vi "RSZVB VI Tree.vi"   [LabVIEW 2011]
doc: "This is the instrument driver for the R&S ZVB Network Analyzer. The VI Tree displays all the user-callable VIs of the instrument driver in an organized table.\n\nInstrument Driver Name: ZVB Network Analyzer\nInstrument Manufacturer: Rohde & Schwarz\nInstrument Type: Network Analyzer\nSupported Models: ZVB Series\nSupported Bus Types: IEEE 488.2 (IEC-625, GPIB), RSIB, VXI-11\n\nInstrument Driver Version: 3.40.0\nSupported Firmware: 3.40\nCreated By: Martin Koutny\nRelease Date: September 2004\nOriginally Developed in LabVIEW Version: 6.1\nOriginally Developed using VISA Version: 3.0.1\n\nUnsupported Instrument Features: none\n\nFor detailed driver information including modification history, refer to the <B>RSZVB.chm </B> file."
panel:
  # "SEE DIAGRAM\nFOR VI TREE."
diagram:
  # "ZVAX-TRM Extension Unit"
  # "Simultaneous Measurement"
  # "Universal Interface"
  # "Get Source Power Calibration Parameters"
  # "Renormalization"
  # "Noise Figure"
  # "Source Power Calibration"
  # "Converter"
  # "Power Port Limits"
  # "PI Controller Low-Level"
  # "Define Port Pair"
  # "Bandwidth Fine Adjust"
  # "Noise Figure"
  # "Low-Level"
  # "Linearity Deviation"
  # "Low Level"
  # "ZVAX Path Configuration"
  # "Low Level"
  # "Pulse Generator"
  # "ZVAX24 Extension Unit"
  # "Fixture Compensation"
  # "Vector Mixer Measurement"
  # "Mixer Delay"
  # "Max Min Hold On"
  # "Defined Coherence Mode"
  # "Intermodulation Distortion"
  # "Multiport Config"
  # "Define Ripple Test"
  # "Ripple"
  # "Power Meter"
  # "True Differential Mode"
  # "Time Out"
  # "Loss Low-Level"
  # "Stimulus"
  # "Pulsed Measurement"
  # "Virtual Transform"
  # "Receiver Power Calibration"
  # "Low-Level"
  # "Modify Source Power Calibration"
  # "Source Power Calibration"
  # "Power Calibration"
  # "Mixer Power Calibration"
  # "Low-Level"
  # "Set Frequencies"
  # "Low-Level"
  # "Set Powers"
  # "Define Mixer Measurement"
  # "Mixer"
  # "System Softkeys"
  # "Low-Level"
  # "Harmonic Distortion"
  # "Define Time Gate"
  # "Low Pass Settings"
  # "Define Transform"
  # "Time Domain Stimulus"
  # "Transform"
  # "Sweep"
  # "Low-Level"
  # "Sweep Time"
  # "Trace Shift"
  # "Import (Export) Data"
  # "Trace Data"
  # "Trace Smoothing"
  # "Trace Evaluation"
  # "User Defined Math"
  # "Define Limit Line(s)"
  # "Status Subsystem"
  # "Initialize"
  # "Close"
  # "Application Example"
  # "Getting Started"
  # "Utility"
  # "Reference"
  # "Channel Bits"
  # "System Config"
  # "System"
  # "Config (View)"
  # "Area Select"
  # "Display"
  # "Mechanical Length Low-Level"
  # "Offset"
  # "Calibration Kits"
  # "Calibration Lists"
  # "Connectors"
  # "Calibration"
  # "Channel Select"
  # "Low-Level"
  # "SAW Matching Network"
  # "Reference Impedances"
  # "Define Balanced Port"
  # "Define Measured Ports"
  # "Port Config"
  # "Mode"
  # "Low-Level"
  # "Trigger"
  # "Define Segments"
  # "Sweep Type"
  # "Low-Level"
  # "Power Bandwidth Average"
  # "Stimulus"
  # "Channel"
  # "Lines"
  # "Marker Funct(ions)"
  # "Bandfilter Search"
  # "Target Search"
  # "Search"
  # "Marker"
  # "Trace Funct(ions)"
  # "Trace Select"
  # "Scale"
  # "Format"
  # "DC Inputs"
  # "Stability Factor"
  # "Y-Parameters"
  # "Z-Parameters"
  # "Admittance"
  # "Impedance"
  # "Wave Quantities"
  # "Ratios"
  # "S-Parameters"
  # "Measure"
  # "Trace"
  # "File (Mass Storage Capabilities)"
  # "Print"
  # "Window Select"
  # "File"
  # "R&S ZVB Network Analyzer"
  n1 = call "RSZVB Set Power Port Limit State.vi"() -> ()  [unwired: 10 in, 2 out]
  n2 = call "RSZVB Set Presets.vi"() -> ()  [unwired: 10 in, 2 out]
  n3 = call "RSZVB Set User Defined Preset State.vi"() -> ()  [unwired: 10 in, 2 out]
  n4 = call "RSZVB Set Display Update.vi"() -> ()  [unwired: 10 in, 2 out]
  n5 = call "RSZVB Get Remote Language.vi"() -> ()  [unwired: 9 in, 3 out]
  n6 = call "RSZVB Configure External Power Meter.vi"() -> ()  [unwired: 10 in, 2 out]
  n7 = call "RSZVB Get Auto Config NRPZxx.vi"() -> ()  [unwired: 9 in, 3 out]
  n8 = call "RSZVB Set Frequency Conversion Type.vi"() -> ()  [unwired: 10 in, 2 out]
  n9 = call "RSZVB Set Power Coeficients.vi"() -> ()  [unwired: 10 in, 2 out]
  n10 = call "RSZVB Set NWA Application Priority.vi"() -> ()  [unwired: 10 in, 2 out]
  n11 = call "RSZVB Set RF Off Behavior.vi"() -> ()  [unwired: 10 in, 2 out]
  n12 = call "RSZVB Set Soft Key Label.vi"() -> ()  [unwired: 10 in, 2 out]
  n13 = call "RSZVB Set Reference.vi"() -> ()  [unwired: 10 in, 2 out]
  n14 = call "RSZVB Set Status Register.vi"() -> ()  [unwired: 10 in, 2 out]
  n15 = call "RSZVB Set Status Sounds State.vi"() -> ()  [unwired: 10 in, 2 out]
  n16 = call "RSZVB Set Output Port Bits.vi"() -> ()  [unwired: 10 in, 2 out]
  n17 = call "RSZVB Set UI Direction.vi"() -> ()  [unwired: 10 in, 2 out]
  n18 = call "RSZVB Set UI Signal Pin 21.vi"() -> ()  [unwired: 10 in, 2 out]
  n19 = call "RSZVB Restore UI Default States.vi"() -> ()  [unwired: 10 in, 2 out]
  n20 = call "RSZVB Reset Offsets.vi"() -> ()  [unwired: 10 in, 2 out]
  n21 = call "RSZVB Configure Loss.vi"() -> ()  [unwired: 10 in, 2 out]
  n22 = call "RSZVB Set Delay.vi"() -> ()  [unwired: 10 in, 2 out]
  n23 = call "RSZVB Set Font Size.vi"() -> ()  [unwired: 10 in, 2 out]
  n24 = call "RSZVB Set RGB Color.vi"() -> ()  [unwired: 10 in, 2 out]
  n25 = call "RSZVB Channel Add.vi"() -> ()  [unwired: 10 in, 2 out]
  n26 = call "RSZVB Channel Get Channel Name.vi"() -> ()  [unwired: 9 in, 3 out]
  n27 = call "RSZVB Diagram Area Add.vi"() -> ()  [unwired: 10 in, 2 out]
  n28 = call "RSZVB Set Color Scheme.vi"() -> ()  [unwired: 10 in, 2 out]
  n29 = call "RSZVB Set Ripple Check On.vi"() -> ()  [unwired: 10 in, 2 out]
  n30 = call "RSZVB Get Ripple Limit Check Segment Result.vi"() -> ()  [unwired: 8 in, 4 out]
  n31 = call "RSZVB Get Number Ripple Limit Ranges.vi"() -> ()  [unwired: 9 in, 3 out]
  n32 = call "RSZVB Set Marker State.vi"() -> ()  [unwired: 10 in, 2 out]
  n33 = call "RSZVB Set Reference Marker State.vi"() -> ()  [unwired: 10 in, 2 out]
  n34 = call "RSZVB Set Reference Discrete Marker.vi"() -> ()  [unwired: 10 in, 2 out]
  n35 = call "RSZVB Get Delta Marker State.vi"() -> ()  [unwired: 9 in, 3 out]
  n36 = call "RSZVB Set Fixed Marker.vi"() -> ()  [unwired: 10 in, 2 out]
  n37 = call "RSZVB Save All Markers.vi"() -> ()  [unwired: 10 in, 2 out]
  n38 = call "RSZVB Trace Get Trace Name.vi"() -> ()  [unwired: 9 in, 3 out]
  n39 = call "RSZVB Set Marker Tracking.vi"() -> ()  [unwired: 10 in, 2 out]
  n40 = call "RSZVB Set Limit Response Domain Format Units.vi"() -> ()  [unwired: 10 in, 2 out]
  n41 = call "RSZVB Window New.vi"() -> ()  [unwired: 10 in, 2 out]
  n42 = call "RSZVB Print.vi"() -> ()  [unwired: 10 in, 2 out]
  n43 = call "RSZVB File Manager.vi"() -> ()  [unwired: 10 in, 2 out]
  n44 = call "RSZVB Setup Recall.vi"() -> ()  [unwired: 10 in, 2 out]
  n45 = call "RSZVB Set Trace Format.vi"() -> ()  [unwired: 10 in, 2 out]
  n46 = call "RSZVB Trace Add.vi"() -> ()  [unwired: 10 in, 2 out]
  n47 = call "RSZVB Trace Add Diagram Area.vi"() -> ()  [unwired: 10 in, 2 out]
  n48 = call "RSZVB Trace Delete All.vi"() -> ()  [unwired: 10 in, 2 out]
  n49 = call "RSZVB Trace Data To Memory.vi"() -> ()  [unwired: 10 in, 2 out]
  n50 = call "RSZVB Marker Search.vi"() -> ()  [unwired: 10 in, 2 out]
  n51 = call "RSZVB Set Start To Marker.vi"() -> ()  [unwired: 10 in, 2 out]
  n52 = call "RSZVB Show Limit Line.vi"() -> ()  [unwired: 10 in, 2 out]
  n53 = call "RSZVB Set Limit Line TTL Out Pass 1(2).vi"() -> ()  [unwired: 10 in, 2 out]
  n54 = call "RSZVB Set Start Frequency.vi"() -> ()  [unwired: 10 in, 2 out]
  n55 = call "RSZVB Set Frequency Span.vi"() -> ()  [unwired: 10 in, 2 out]
  n56 = call "RSZVB Set Start Power.vi"() -> ()  [unwired: 10 in, 2 out]
  n57 = call "RSZVB Configure Power Bandwidth Average.vi"() -> ()  [unwired: 10 in, 2 out]
  n58 = call "RSZVB Get Trace Ref Position.vi"() -> ()  [unwired: 9 in, 3 out]
  n59 = call "RSZVB Trace Autoscale.vi"() -> ()  [unwired: 10 in, 2 out]
  n60 = call "RSZVB Get Trace Scale Divisions.vi"() -> ()  [unwired: 9 in, 3 out]
  n61 = call "RSZVB Create Trace.vi"() -> ()  [unwired: 10 in, 2 out]
  n62 = call "RSZVB Set Loss At DC.vi"() -> ()  [unwired: 10 in, 2 out]
  n63 = call "RSZVB Get Delay.vi"() -> ()  [unwired: 9 in, 3 out]
  n64 = call "RSZVB Acquire Fixture Compensation Sweep.vi"() -> ()  [unwired: 10 in, 2 out]
  n65 = call "RSZVB Set Fixture Compensation Direct Compensation.vi"() -> ()  [unwired: 10 in, 2 out]
  n66 = call "RSZVB Get Power Port Limit State.vi"() -> ()  [unwired: 9 in, 3 out]
  n67 = call "RSZVB Get Presets.vi"() -> ()  [unwired: 9 in, 3 out]
  n68 = call "RSZVB Get Display Update.vi"() -> ()  [unwired: 9 in, 3 out]
  n69 = call "RSZVB Configure External Generator.vi"() -> ()  [unwired: 14 in, 2 out]
  n70 = call "RSZVB Query External Power Meter.vi"() -> ()  [unwired: 6 in, 6 out]
  n71 = call "RSZVB Delete External Power Meter.vi"() -> ()  [unwired: 10 in, 2 out]
  n72 = call "RSZVB Get Status Sounds State.vi"() -> ()  [unwired: 9 in, 3 out]
  n73 = call "RSZVB Get Frequency Conversion Type.vi"() -> ()  [unwired: 9 in, 3 out]
  n74 = call "RSZVB Get Power Coeficients.vi"() -> ()  [unwired: 9 in, 3 out]
  n75 = call "RSZVB Get NWA Application Priority.vi"() -> ()  [unwired: 9 in, 3 out]
  n76 = call "RSZVB Get RF Off Behavior.vi"() -> ()  [unwired: 9 in, 3 out]
  n77 = call "RSZVB Get Pressed Soft Key.vi"() -> ()  [unwired: 8 in, 4 out]
  n78 = call "RSZVB Get Output Port Bits.vi"() -> ()  [unwired: 9 in, 3 out]
  n79 = call "RSZVB Get UI Direction.vi"() -> ()  [unwired: 9 in, 3 out]
  n80 = call "RSZVB Get UI Signal Pin 21.vi"() -> ()  [unwired: 9 in, 3 out]
  n81 = call "RSZVB Get Reference.vi"() -> ()  [unwired: 9 in, 3 out]
  n82 = call "RSZVB Get Status Register.vi"() -> ()  [unwired: 9 in, 3 out]
  n83 = call "RSZVB Set Mechanical Length.vi"() -> ()  [unwired: 10 in, 2 out]
  n84 = call "RSZVB Get RGB Color.vi"() -> ()  [unwired: 5 in, 7 out]
  n85 = call "RSZVB Get User Defined Preset State.vi"() -> ()  [unwired: 9 in, 3 out]
  n86 = call "RSZVB Export Kit.vi"() -> ()  [unwired: 10 in, 2 out]
  n87 = call "RSZVB Channel Add Trace.vi"() -> ()  [unwired: 10 in, 2 out]
  n88 = call "RSZVB Channel Get Channel Number.vi"() -> ()  [unwired: 9 in, 3 out]
  n89 = call "RSZVB Set Connector.vi"() -> ()  [unwired: 10 in, 2 out]
  n90 = call "RSZVB Select Calibration Type.vi"() -> ()  [unwired: 14 in, 2 out]
  n91 = call "RSZVB Get Calibration Reference Plane Shift.vi"() -> ()  [unwired: 9 in, 3 out]
  n92 = call "RSZVB Delete Calibration Data.vi"() -> ()  [unwired: 10 in, 2 out]
  n93 = call "RSZVB Set Calibration Kit.vi"() -> ()  [unwired: 10 in, 2 out]
  n94 = call "RSZVB Calibration Kit Catalog With Label.vi"() -> ()  [unwired: 9 in, 3 out]
  n95 = call "RSZVB Load Calibration Kit.vi"() -> ()  [unwired: 14 in, 2 out]
  n96 = call "RSZVB Query Reset Offsets.vi"() -> ()  [unwired: 9 in, 3 out]
  n97 = call "RSZVB Diagram Area Delete.vi"() -> ()  [unwired: 10 in, 2 out]
  n98 = call "RSZVB Get Color Scheme.vi"() -> ()  [unwired: 9 in, 3 out]
  n99 = call "RSZVB Get Font Size.vi"() -> ()  [unwired: 9 in, 3 out]
  n100 = call "RSZVB Set User Connector.vi"() -> ()  [unwired: 10 in, 2 out]
  n101 = call "RSZVB Set Source Power Correction State.vi"() -> ()  [unwired: 10 in, 2 out]
  n102 = call "RSZVB Calibration Auto Simplified.vi"() -> ()  [unwired: 10 in, 2 out]
  n103 = call "RSZVB Calibration Auto Assignment Type.vi"() -> ()  [unwired: 10 in, 2 out]
  n104 = call "RSZVB Set Calibration Data Current State.vi"() -> ()  [unwired: 10 in, 2 out]
  n105 = call "RSZVB Set Calibration Connector.vi"() -> ()  [unwired: 10 in, 2 out]
  n106 = call "RSZVB Get Calibration Label.vi"() -> ()  [unwired: 9 in, 3 out]
  n107 = call "RSZVB Get Calibration Data Receiver Attenuation.vi"() -> ()  [unwired: 8 in, 4 out]
  n108 = call "RSZVB Get Active Calibration Unit.vi"() -> ()  [unwired: 9 in, 3 out]
  n109 = call "RSZVB Get Factory Calibration State.vi"() -> ()  [unwired: 9 in, 3 out]
  n110 = call "RSZVB Get Calibration Correction Base Frequency State.vi"() -> ()  [unwired: 9 in, 3 out]
  n111 = call "RSZVB Get Ripple Check On.vi"() -> ()  [unwired: 9 in, 3 out]
  n112 = call "RSZVB Set Ripple Limits Display State.vi"() -> ()  [unwired: 10 in, 2 out]
  n113 = call "RSZVB Add Ripple Limit Line Ranges Segment.vi"() -> ()  [unwired: 10 in, 2 out]
  n114 = call "RSZVB Set Ripple Limit Range.vi"() -> ()  [unwired: 10 in, 2 out]
  n115 = call "RSZVB Get Marker Tracking.vi"() -> ()  [unwired: 9 in, 3 out]
  n116 = call "RSZVB Set Sweep Number Of Points.vi"() -> ()  [unwired: 10 in, 2 out]
  n117 = call "RSZVB Configure Sweep Time.vi"() -> ()  [unwired: 10 in, 2 out]
  n118 = call "RSZVB Trace Add Mode.vi"() -> ()  [unwired: 10 in, 2 out]
  n119 = call "RSZVB Trace Assign Diagram Area.vi"() -> ()  [unwired: 10 in, 2 out]
  n120 = call "RSZVB Channel Trace Export Data With Options.vi"() -> ()  [unwired: 10 in, 2 out]
  n121 = call "RSZVB Set Coherent Signal Reference Port.vi"() -> ()  [unwired: 10 in, 2 out]
  n122 = call "RSZVB Trace Delete All Channels.vi"() -> ()  [unwired: 10 in, 2 out]
  n123 = call "RSZVB Trace Get Trace Number.vi"() -> ()  [unwired: 9 in, 3 out]
  n124 = call "RSZVB Trace Data To Memory Trace.vi"() -> ()  [unwired: 10 in, 2 out]
  n125 = call "RSZVB Get Marker State.vi"() -> ()  [unwired: 9 in, 3 out]
  n126 = call "RSZVB Get Reference Marker State.vi"() -> ()  [unwired: 9 in, 3 out]
  n127 = call "RSZVB Get Reference Discrete Marker.vi"() -> ()  [unwired: 9 in, 3 out]
  n128 = call "RSZVB Set Coupled Markers.vi"() -> ()  [unwired: 10 in, 2 out]
  n129 = call "RSZVB Get Fixed Marker.vi"() -> ()  [unwired: 9 in, 3 out]
  n130 = call "RSZVB Set Frequency Conversion.vi"() -> ()  [unwired: 14 in, 2 out]
  n131 = call "RSZVB Set Converter Source Frequency.vi"() -> ()  [unwired: 10 in, 2 out]
  n132 = call "RSZVB Set Local Oscilator B State.vi"() -> ()  [unwired: 10 in, 2 out]
  n133 = call "RSZVB Set Port Impedances Renormalization.vi"() -> ()  [unwired: 10 in, 2 out]
  n134 = call "RSZVB Set IF Gain Reference Channel.vi"() -> ()  [unwired: 10 in, 2 out]
  n135 = call "RSZVB Set Permanent Signal Generator State.vi"() -> ()  [unwired: 10 in, 2 out]
  n136 = call "RSZVB Set Source Combiner State.vi"() -> ()  [unwired: 10 in, 2 out]
  n137 = call "RSZVB Set TDIF State.vi"() -> ()  [unwired: 10 in, 2 out]
  n138 = call "RSZVB Get TDIF Amplitude Imbalance Start Power.vi"() -> ()  [unwired: 9 in, 3 out]
  n139 = call "RSZVB Set TDIF Phase Imbalance Start Phase.vi"() -> ()  [unwired: 10 in, 2 out]
  n140 = call "RSZVB Get TDIF Source Power Mode.vi"() -> ()  [unwired: 9 in, 3 out]
  n141 = call "RSZVB Set TRM Measure Input.vi"() -> ()  [unwired: 10 in, 2 out]
  n142 = call "RSZVB Get TRM Power Amplifier State.vi"() -> ()  [unwired: 9 in, 3 out]
  n143 = call "RSZVB Set TRM User Measurement Path Extension State.vi"() -> ()  [unwired: 10 in, 2 out]
  n144 = call "RSZVB Get TRM Pulse Generator Source.vi"() -> ()  [unwired: 9 in, 3 out]
  n145 = call "RSZVB Get TRM Unit Hardware Options.vi"() -> ()  [unwired: 9 in, 3 out]
  n146 = call "RSZVB Configure Harmonic Measurement.vi"() -> ()  [unwired: 10 in, 2 out]
  n147 = call "RSZVB Set Mixer Mode.vi"() -> ()  [unwired: 10 in, 2 out]
  n148 = call "RSZVB Set Coherent Signal State.vi"() -> ()  [unwired: 10 in, 2 out]
  n149 = call "RSZVB Set Alternate Sweep Mode.vi"() -> ()  [unwired: 10 in, 2 out]
  n150 = call "RSZVB Set Individual ALC Port State.vi"() -> ()  [unwired: 10 in, 2 out]
  n151 = call "RSZVB Set ALC Port AUBW State.vi"() -> ()  [unwired: 10 in, 2 out]
  n152 = call "RSZVB Set ALC Channel State.vi"() -> ()  [unwired: 10 in, 2 out]
  n153 = call "RSZVB Set ALC Port Control Range.vi"() -> ()  [unwired: 10 in, 2 out]
  n154 = call "RSZVB Set Low Phase Noise State.vi"() -> ()  [unwired: 10 in, 2 out]
  n155 = call "RSZVB Configure SAW Matching Network.vi"() -> ()  [unwired: 10 in, 2 out]
  n156 = call "RSZVB Trace User Defined Math.vi"() -> ()  [unwired: 10 in, 2 out]
  n157 = call "RSZVB Set Trace Transform Domain.vi"() -> ()  [unwired: 10 in, 2 out]
  n158 = call "RSZVB Set Time Gate State.vi"() -> ()  [unwired: 10 in, 2 out]
  n159 = call "RSZVB Set Time Gate Start Time.vi"() -> ()  [unwired: 10 in, 2 out]
  n160 = call "RSZVB Get Time Gate Center Time.vi"() -> ()  [unwired: 9 in, 3 out]
  n161 = call "RSZVB Set Time Gate Sideband Suppression.vi"() -> ()  [unwired: 10 in, 2 out]
  n162 = call "RSZVB Get Time Gate Span.vi"() -> ()  [unwired: 9 in, 3 out]
  n163 = call "RSZVB Trace Evaluation Range.vi"() -> ()  [unwired: 10 in, 2 out]
  n164 = call "RSZVB Get Trace Compression Value.vi"() -> ()  [unwired: 9 in, 3 out]
  n165 = call "RSZVB Set Trace Smoothing.vi"() -> ()  [unwired: 10 in, 2 out]
  n166 = call "RSZVB Trace Response Data.vi"() -> ()  [unwired: 9 in, 3 out]
  n167 = call "RSZVB Trace Response Data All Data.vi"() -> ()  [unwired: 9 in, 3 out]
  n168 = call "RSZVB Set Trace Format ZVR.vi"() -> ()  [unwired: 10 in, 2 out]
  n169 = call "RSZVB Trace Import Data.vi"() -> ()  [unwired: 10 in, 2 out]
  n170 = call "RSZVB Trace Shift Stimulus Value.vi"() -> ()  [unwired: 10 in, 2 out]
  n171 = call "RSZVB Set Hold.vi"() -> ()  [unwired: 10 in, 2 out]
  n172 = call "RSZVB Linearity Deviation Manual.vi"() -> ()  [unwired: 10 in, 2 out]
  n173 = call "RSZVB Set Sweep Type.vi"() -> ()  [unwired: 10 in, 2 out]
  n174 = call "RSZVB Send Trigger.vi"() -> ()  [unwired: 10 in, 2 out]
  n175 = call "RSZVB Set IMOD Lower Tone Source.vi"() -> ()  [unwired: 10 in, 2 out]
  n176 = call "RSZVB Set IMOD Enhanced Wave Correction.vi"() -> ()  [unwired: 10 in, 2 out]
  n177 = call "RSZVB Set Noise Figure Detector Measurement Time.vi"() -> ()  [unwired: 10 in, 2 out]
  n178 = call "RSZVB Set Noise Figure Narowband DUT.vi"() -> ()  [unwired: 10 in, 2 out]
  n179 = call "RSZVB Get Noise Figure Calibration State Label.vi"() -> ()  [unwired: 9 in, 3 out]
  n180 = call "RSZVB Set Virtual Transform Balanced State.vi"() -> ()  [unwired: 10 in, 2 out]
  n181 = call "RSZVB Load Balanced Port Circuit Model Data.vi"() -> ()  [unwired: 10 in, 2 out]
  n182 = call "RSZVB Set Virtual Transform Single Ended Circuit Model.vi"() -> ()  [unwired: 10 in, 2 out]
  n183 = call "RSZVB Set Virtual Transform Ground Loop.vi"() -> ()  [unwired: 10 in, 2 out]
  n184 = call "RSZVB Get Virtual Transform Port Pair State.vi"() -> ()  [unwired: 9 in, 3 out]
  n185 = call "RSZVB Read To File From Instrument.vi"() -> ()  [unwired: 10 in, 2 out]
  n186 = call "RSZVB Select Power Meter.vi"() -> ()  [unwired: 10 in, 2 out]
  n187 = call "RSZVB Select S-Parameters.vi"() -> ()  [unwired: 10 in, 2 out]
  n188 = call "RSZVB Select Ratios.vi"() -> ()  [unwired: 10 in, 2 out]
  n189 = call "RSZVB Select Wave Quantities.vi"() -> ()  [unwired: 10 in, 2 out]
  n190 = call "RSZVB Select Impedances.vi"() -> ()  [unwired: 10 in, 2 out]
  n191 = call "RSZVB Select Admitances.vi"() -> ()  [unwired: 10 in, 2 out]
  n192 = call "RSZVB Select Z-Parameters.vi"() -> ()  [unwired: 10 in, 2 out]
  n193 = call "RSZVB Select Y-Parameters.vi"() -> ()  [unwired: 10 in, 2 out]
  n194 = call "RSZVB Select Stability Factors.vi"() -> ()  [unwired: 10 in, 2 out]
  n195 = call "RSZVB Select DC Measurement.vi"() -> ()  [unwired: 10 in, 2 out]
  n196 = call "RSZVB Select Noise Figure.vi"() -> ()  [unwired: 10 in, 2 out]
  n197 = call "RSZVB Get Trace Format.vi"() -> ()  [unwired: 9 in, 3 out]
  n198 = call "RSZVB Marker Target Search.vi"() -> ()  [unwired: 10 in, 2 out]
  n199 = call "RSZVB Marker Bandpass Search.vi"() -> ()  [unwired: 10 in, 2 out]
  n200 = call "RSZVB Marker x dB Bandwidth.vi"() -> ()  [unwired: 10 in, 2 out]
  n201 = call "RSZVB Get Marker Search Result State.vi"() -> ()  [unwired: 9 in, 3 out]
  n202 = call "RSZVB Set Stop To Marker.vi"() -> ()  [unwired: 10 in, 2 out]
  n203 = call "RSZVB Set Limit Check.vi"() -> ()  [unwired: 10 in, 2 out]
  n204 = call "RSZVB Add Limit Line Segment.vi"() -> ()  [unwired: 14 in, 2 out]
  n205 = call "RSZVB Delete Limit Line Segments.vi"() -> ()  [unwired: 10 in, 2 out]
  n206 = call "RSZVB Get Limit Line TTL Out Pass 1(2).vi"() -> ()  [unwired: 9 in, 3 out]
  n207 = call "RSZVB Set Limit Response Domain Spacing Units.vi"() -> ()  [unwired: 10 in, 2 out]
  n208 = call "RSZVB Get Start Frequency.vi"() -> ()  [unwired: 9 in, 3 out]
  n209 = call "RSZVB Get Frequency Span.vi"() -> ()  [unwired: 9 in, 3 out]
  n210 = call "RSZVB Get Start Power.vi"() -> ()  [unwired: 9 in, 3 out]
  n211 = call "RSZVB Set Partial Measurement Resolution Bandwidth Mode.vi"() -> ()  [unwired: 10 in, 2 out]
  n212 = call "RSZVB Sweep Restart.vi"() -> ()  [unwired: 10 in, 2 out]
  n213 = call "RSZVB Set IMOD Max Order.vi"() -> ()  [unwired: 10 in, 2 out]
  n214 = call "RSZVB Start IMOD Receiver Port Power Calibration.vi"() -> ()  [unwired: 10 in, 2 out]
  n215 = call "RSZVB Set PI Controller Mode.vi"() -> ()  [unwired: 10 in, 2 out]
  n216 = call "RSZVB Window Select.vi"() -> ()  [unwired: 10 in, 2 out]
  n217 = call "RSZVB Print to File.vi"() -> ()  [unwired: 10 in, 2 out]
  n218 = call "RSZVB Get Current Directory.vi"() -> ()  [unwired: 9 in, 3 out]
  n219 = call "RSZVB Configure Measurement Parameters.vi"() -> ()  [unwired: 10 in, 2 out]
  n220 = call "RSZVB Set Receiver Step Attenuators.vi"() -> ()  [unwired: 10 in, 2 out]
  n221 = call "RSZVB Get Automatic Generator Attenuation.vi"() -> ()  [unwired: 9 in, 3 out]
  n222 = call "RSZVB Get Meas Bandwidth.vi"() -> ()  [unwired: 9 in, 3 out]
  n223 = call "RSZVB Get Average State.vi"() -> ()  [unwired: 9 in, 3 out]
  n224 = call "RSZVB Configure Trigger Free Run.vi"() -> ()  [unwired: 10 in, 2 out]
  n225 = call "RSZVB Trace Autoscale By Name.vi"() -> ()  [unwired: 10 in, 2 out]
  n226 = call "RSZVB Set Trace Ref Value.vi"() -> ()  [unwired: 10 in, 2 out]
  n227 = call "RSZVB Set Trace Top.vi"() -> ()  [unwired: 10 in, 2 out]
  n228 = call "RSZVB Set Channel Bits.vi"() -> ()  [unwired: 10 in, 2 out]
  n229 = call "RSZVB Set UI Data.vi"() -> ()  [unwired: 10 in, 2 out]
  n230 = call "RSZVB Set UI Port Binary Data.vi"() -> ()  [unwired: 10 in, 2 out]
  n231 = call "RSZVB Set Reference Frequency.vi"() -> ()  [unwired: 10 in, 2 out]
  n232 = call "RSZVB Set Pulse Generator State.vi"() -> ()  [unwired: 10 in, 2 out]
  n233 = call "RSZVB Configure ZVAX Path.vi"() -> ()  [unwired: 10 in, 2 out]
  n234 = call "RSZVB Set Power Port Limit Value.vi"() -> ()  [unwired: 10 in, 2 out]
  n235 = call "RSZVB Set Preset Settings State.vi"() -> ()  [unwired: 10 in, 2 out]
  n236 = call "RSZVB Immediate Settings Update.vi"() -> ()  [unwired: 10 in, 2 out]
  n237 = call "RSZVB Query External Generator.vi"() -> ()  [unwired: 8 in, 8 out]
  n238 = call "RSZVB Query External Power Meter Count.vi"() -> ()  [unwired: 9 in, 3 out]
  n239 = call "RSZVB Set Alarm Sounds State.vi"() -> ()  [unwired: 10 in, 2 out]
  n240 = call "RSZVB Set Data Transfer.vi"() -> ()  [unwired: 10 in, 2 out]
  n241 = call "RSZVB Set Frequency Conversion Source.vi"() -> ()  [unwired: 10 in, 2 out]
  n242 = call "RSZVB Set Power Coeficients Default.vi"() -> ()  [unwired: 10 in, 2 out]
  n243 = call "RSZVB System Shutdown.vi"() -> ()  [unwired: 10 in, 2 out]
  n244 = call "RSZVB Set Remote Display Title.vi"() -> ()  [unwired: 10 in, 2 out]
  n245 = call "RSZVB Set User Defined Preset File.vi"() -> ()  [unwired: 10 in, 2 out]
  n246 = call "RSZVB Set B Wave Receiver Power Calibration State.vi"() -> ()  [unwired: 10 in, 2 out]
  n247 = call "RSZVB Set Calibration Kit Label.vi"() -> ()  [unwired: 10 in, 2 out]
  n248 = call "RSZVB Export Kit With Label.vi"() -> ()  [unwired: 10 in, 2 out]
  n249 = call "RSZVB Get Mechanical Length.vi"() -> ()  [unwired: 9 in, 3 out]
  n250 = call "RSZVB Save Color Scheme.vi"() -> ()  [unwired: 10 in, 2 out]
  n251 = call "RSZVB Set Channel Info.vi"() -> ()  [unwired: 10 in, 2 out]
  n252 = call "RSZVB Set Trace Color State.vi"() -> ()  [unwired: 10 in, 2 out]
  n253 = call "RSZVB Set Source Power Calibration Port State.vi"() -> ()  [unwired: 10 in, 2 out]
  n254 = call "RSZVB Set Verification Sweep State.vi"() -> ()  [unwired: 10 in, 2 out]
  n255 = call "RSZVB Set Source Power Calibration State.vi"() -> ()  [unwired: 10 in, 2 out]
  n256 = call "RSZVB Read Source Power Correction Data.vi"() -> ()  [unwired: 9 in, 3 out]
  n257 = call "RSZVB Set Source Power Calibration Converter State.vi"() -> ()  [unwired: 10 in, 2 out]
  n258 = call "RSZVB Acquire Receiver Power Calibration.vi"() -> ()  [unwired: 10 in, 2 out]
  n259 = call "RSZVB Correction Manager.vi"() -> ()  [unwired: 10 in, 2 out]
  n260 = call "RSZVB Get Two Port Transmission Coefficients Enabled.vi"() -> ()  [unwired: 9 in, 3 out]
  n261 = call "RSZVB Delete All Power Loss List Points.vi"() -> ()  [unwired: 10 in, 2 out]
  n262 = call "RSZVB Get Source Power Correction State.vi"() -> ()  [unwired: 9 in, 3 out]
  n263 = call "RSZVB Get Calibration Kit.vi"() -> ()  [unwired: 9 in, 3 out]
  n264 = call "RSZVB Import ZVR Calibration Kit.vi"() -> ()  [unwired: 10 in, 2 out]
  n265 = call "RSZVB Get Loss At DC.vi"() -> ()  [unwired: 9 in, 3 out]
  n266 = call "RSZVB Query Direct Fixture Compensation.vi"() -> ()  [unwired: 9 in, 3 out]
  n267 = call "RSZVB Start Fixture Compensation Sweep.vi"() -> ()  [unwired: 10 in, 2 out]
  n268 = call "RSZVB Get Fixture Compensation Direct Compensation.vi"() -> ()  [unwired: 9 in, 3 out]
  n269 = call "RSZVB Diagram Area Maximize.vi"() -> ()  [unwired: 10 in, 2 out]
  n270 = call "RSZVB Get User Connector.vi"() -> ()  [unwired: 8 in, 4 out]
  n271 = call "RSZVB Acquire Source Power Calibration.vi"() -> ()  [unwired: 10 in, 2 out]
  n272 = call "RSZVB Get Calibration Connector.vi"() -> ()  [unwired: 6 in, 6 out]
  n273 = call "RSZVB Get Calibration Data Parameters.vi"() -> ()  [unwired: 9 in, 7 out]
  n274 = call "RSZVB Get Calibration Data Type.vi"() -> ()  [unwired: 9 in, 3 out]
  n275 = call "RSZVB Set Automatic Power Reduction State.vi"() -> ()  [unwired: 10 in, 2 out]
  n276 = call "RSZVB Initialize.vi"() -> ()  [unwired: 10 in, 2 out]
  n277 = call "RSZVB Calibration Auto Type.vi"() -> ()  [unwired: 18 in, 2 out]
  n278 = call "RSZVB Calibration Auto Assignment Definition.vi"() -> ()  [unwired: 14 in, 2 out]
  n279 = call "RSZVB Get Calibration Data Current State.vi"() -> ()  [unwired: 9 in, 3 out]
  n280 = call "RSZVB Set Enhanced Wave Correction.vi"() -> ()  [unwired: 10 in, 2 out]
  n281 = call "RSZVB Set Electrical Length.vi"() -> ()  [unwired: 10 in, 2 out]
  n282 = call "RSZVB Channel Add Trace Diagram Area.vi"() -> ()  [unwired: 10 in, 2 out]
  n283 = call "RSZVB Channel Set Active.vi"() -> ()  [unwired: 10 in, 2 out]
  n284 = call "RSZVB Get Connector.vi"() -> ()  [unwired: 9 in, 3 out]
  n285 = call "RSZVB Get Calibration Type.vi"() -> ()  [unwired: 9 in, 7 out]
  n286 = call "RSZVB Set Calibration Reference Plane Shift Specific.vi"() -> ()  [unwired: 10 in, 2 out]
  n287 = call "RSZVB Delete All Calibration Data.vi"() -> ()  [unwired: 10 in, 2 out]
  n288 = call "RSZVB Insert New Segment.vi"() -> ()  [unwired: 18 in, 2 out]
  n289 = call "RSZVB Set Sweep Segment State.vi"() -> ()  [unwired: 10 in, 2 out]
  n290 = call "RSZVB Set Sweep Segment Number Of Points.vi"() -> ()  [unwired: 10 in, 2 out]
  n291 = call "RSZVB Set Sweep Segment Independent Power.vi"() -> ()  [unwired: 10 in, 2 out]
  n292 = call "RSZVB Set Sweep Segment Spur Avoid.vi"() -> ()  [unwired: 10 in, 2 out]
  n293 = call "RSZVB Set Sweep Segment Independent Selectivity.vi"() -> ()  [unwired: 10 in, 2 out]
  n294 = call "RSZVB Set Sweep Segment Point Delay.vi"() -> ()  [unwired: 10 in, 2 out]
  n295 = call "RSZVB Set Sweep Selective Segment Triggering.vi"() -> ()  [unwired: 10 in, 2 out]
  n296 = call "RSZVB Get Sweep Segment Center Frequency.vi"() -> ()  [unwired: 9 in, 3 out]
  n297 = call "RSZVB Marker Search Range.vi"() -> ()  [unwired: 10 in, 2 out]
  n298 = call "RSZVB Get Ripple Limit Global Check Result.vi"() -> ()  [unwired: 9 in, 3 out]
  n299 = call "RSZVB Get Ripple Limits Display State.vi"() -> ()  [unwired: 9 in, 3 out]
  n300 = call "RSZVB Edit Ripple Limit Line Segment.vi"() -> ()  [unwired: 10 in, 2 out]
  n301 = call "RSZVB Get Ripple Limit Range.vi"() -> ()  [unwired: 9 in, 3 out]
  n302 = call "RSZVB Set Pulse Time Start.vi"() -> ()  [unwired: 10 in, 2 out]
  n303 = call "RSZVB Set Pulse Coupled Section Limit Lines State.vi"() -> ()  [unwired: 10 in, 2 out]
  n304 = call "RSZVB Set Pulse Evaluation Section Stop.vi"() -> ()  [unwired: 10 in, 2 out]
  n305 = call "RSZVB Read Time Samples Data.vi"() -> ()  [unwired: 9 in, 3 out]
  n306 = call "RSZVB Get Trace Compression Point.vi"() -> ()  [unwired: 8 in, 4 out]
  n307 = call "RSZVB Set Renormalization Impedance.vi"() -> ()  [unwired: 10 in, 2 out]
  n308 = call "RSZVB Set Sweep Time.vi"() -> ()  [unwired: 10 in, 2 out]
  n309 = call "RSZVB Set Frequency Stimulus.vi"() -> ()  [unwired: 10 in, 2 out]
  n310 = call "RSZVB Set Harmonic Measurement State.vi"() -> ()  [unwired: 10 in, 2 out]
  n311 = call "RSZVB Get Harmonic Source Port.vi"() -> ()  [unwired: 9 in, 3 out]
  n312 = call "RSZVB Get Mixer Mode.vi"() -> ()  [unwired: 9 in, 3 out]
  n313 = call "RSZVB Get PI Controller Mode.vi"() -> ()  [unwired: 9 in, 3 out]
  n314 = call "RSZVB Set Renormalization State.vi"() -> ()  [unwired: 10 in, 2 out]
  n315 = call "RSZVB Get Sweep Number Of Points.vi"() -> ()  [unwired: 9 in, 3 out]
  n316 = call "RSZVB Set External Power Meter.vi"() -> ()  [unwired: 10 in, 2 out]
  n317 = call "RSZVB Set Mixer Delay Measurement Setup.vi"() -> ()  [unwired: 10 in, 2 out]
  n318 = call "RSZVB Clear Mixer Delay Receiver List.vi"() -> ()  [unwired: 10 in, 2 out]
  n319 = call "RSZVB Get Mixer Delay Constant.vi"() -> ()  [unwired: 9 in, 3 out]
  n320 = call "RSZVB Set Mixer Constant Delay Enabled.vi"() -> ()  [unwired: 10 in, 2 out]
  n321 = call "RSZVB Set Vector Mixer Mode.vi"() -> ()  [unwired: 10 in, 2 out]
  n322 = call "RSZVB Get External Signal Source AUX.vi"() -> ()  [unwired: 9 in, 3 out]
  n323 = call "RSZVB Get Alternate Sweep Mode.vi"() -> ()  [unwired: 9 in, 3 out]
  n324 = call "RSZVB Get Individual ALC Port State.vi"() -> ()  [unwired: 9 in, 3 out]
  n325 = call "RSZVB Get ALC Port AUBW State.vi"() -> ()  [unwired: 9 in, 3 out]
  n326 = call "RSZVB Get ALC Channel State.vi"() -> ()  [unwired: 9 in, 3 out]
  n327 = call "RSZVB Get ALC Port Control Range.vi"() -> ()  [unwired: 9 in, 3 out]
  n328 = call "RSZVB Set SAW State.vi"() -> ()  [unwired: 10 in, 2 out]
  n329 = call "RSZVB Get SAW Serial C.vi"() -> ()  [unwired: 9 in, 3 out]
  n330 = call "RSZVB Set Trace Display State.vi"() -> ()  [unwired: 10 in, 2 out]
  n331 = call "RSZVB Trace Assign Window Diagram Area.vi"() -> ()  [unwired: 10 in, 2 out]
  n332 = call "RSZVB Trace List.vi"() -> ()  [unwired: 9 in, 3 out]
  n333 = call "RSZVB Trace Get Channel Name.vi"() -> ()  [unwired: 9 in, 3 out]
  n334 = call "RSZVB Trace Math To Memory Trace.vi"() -> ()  [unwired: 10 in, 2 out]
  n335 = call "RSZVB Channel Trace Export Data With Options Extended.vi"() -> ()  [unwired: 14 in, 2 out]
  n336 = call "RSZVB Get Sweep Type.vi"() -> ()  [unwired: 9 in, 3 out]
  n337 = call "RSZVB Set RF Signal Port.vi"() -> ()  [unwired: 10 in, 2 out]
  n338 = call "RSZVB Get Mixer Delay Upper Tone Source.vi"() -> ()  [unwired: 8 in, 4 out]
  n339 = call "RSZVB Get Coherent Signal State.vi"() -> ()  [unwired: 9 in, 3 out]
  n340 = call "RSZVB Get Coherent Signal Reference Port.vi"() -> ()  [unwired: 9 in, 3 out]
  n341 = call "RSZVB Get Low Phase Noise State.vi"() -> ()  [unwired: 9 in, 3 out]
  n342 = call "RSZVB Trace Export Data.vi"() -> ()  [unwired: 10 in, 2 out]
  n343 = call "RSZVB Trace Shift Response Value.vi"() -> ()  [unwired: 10 in, 2 out]
  n344 = call "RSZVB Get Hold.vi"() -> ()  [unwired: 9 in, 3 out]
  n345 = call "RSZVB Linearity Deviation Auto.vi"() -> ()  [unwired: 10 in, 2 out]
  n346 = call "RSZVB Set Linearity Deviation Slope.vi"() -> ()  [unwired: 10 in, 2 out]
  n347 = call "RSZVB Set Default Configuration State.vi"() -> ()  [unwired: 10 in, 2 out]
  n348 = call "RSZVB Set Pulse Generator Type.vi"() -> ()  [unwired: 10 in, 2 out]
  n349 = call "RSZVB Set Pulse Generator Polarity.vi"() -> ()  [unwired: 10 in, 2 out]
  n350 = call "RSZVB Get Pulse Train Segment State.vi"() -> ()  [unwired: 9 in, 3 out]
  n351 = call "RSZVB Load Pulse Train File.vi"() -> ()  [unwired: 10 in, 2 out]
  n352 = call "RSZVB Set Number Of Stages.vi"() -> ()  [unwired: 10 in, 2 out]
  n353 = call "RSZVB Get Time Gate Start Time.vi"() -> ()  [unwired: 9 in, 3 out]
  n354 = call "RSZVB Set Time Gate Type.vi"() -> ()  [unwired: 10 in, 2 out]
  n355 = call "RSZVB Get Time Gate Sideband Suppression.vi"() -> ()  [unwired: 9 in, 3 out]
  n356 = call "RSZVB Set Time Gate Display State.vi"() -> ()  [unwired: 10 in, 2 out]
  n357 = call "RSZVB Trace Statistical Evaluation.vi"() -> ()  [unwired: 9 in, 3 out]
  n358 = call "RSZVB Trace Response Data Error.vi"() -> ()  [unwired: 9 in, 3 out]
  n359 = call "RSZVB Trace Response Single Sweep Data Count.vi"() -> ()  [unwired: 9 in, 3 out]
  n360 = call "RSZVB Get Trace Format ZVR.vi"() -> ()  [unwired: 9 in, 3 out]
  n361 = call "RSZVB Set Marker Stimulus.vi"() -> ()  [unwired: 10 in, 2 out]
  n362 = call "RSZVB Set Reference Marker Stimulus.vi"() -> ()  [unwired: 10 in, 2 out]
  n363 = call "RSZVB Set Reference Fixed Marker.vi"() -> ()  [unwired: 10 in, 2 out]
  n364 = call "RSZVB Get Coupled Markers.vi"() -> ()  [unwired: 9 in, 3 out]
  n365 = call "RSZVB Set Marker Format.vi"() -> ()  [unwired: 10 in, 2 out]
  n366 = call "RSZVB Marker Bandfilter Results.vi"() -> ()  [unwired: 8 in, 8 out]
  n367 = call "RSZVB Configure Trigger External.vi"() -> ()  [unwired: 10 in, 2 out]
  n368 = call "RSZVB Set Trigger Source.vi"() -> ()  [unwired: 10 in, 2 out]
  n369 = call "RSZVB Get Partial Measurement Trigger Mode.vi"() -> ()  [unwired: 9 in, 3 out]
  n370 = call "RSZVB Set Triggered Meas Sequence.vi"() -> ()  [unwired: 10 in, 2 out]
  n371 = call "RSZVB Get Trigger Period.vi"() -> ()  [unwired: 9 in, 3 out]
  n372 = call "RSZVB Send Channel Trigger and Wait for OPC.vi"() -> ()  [unwired: 10 in, 2 out]
  n373 = call "RSZVB Set Sweep Single.vi"() -> ()  [unwired: 10 in, 2 out]
  n374 = call "RSZVB Define Group Of Measured Ports.vi"() -> ()  [unwired: 10 in, 2 out]
  n375 = call "RSZVB Delete All Groups Of Measured Ports.vi"() -> ()  [unwired: 10 in, 2 out]
  n376 = call "RSZVB Define Balanced Port.vi"() -> ()  [unwired: 10 in, 2 out]
  n377 = call "RSZVB Get Frequency Conversion.vi"() -> ()  [unwired: 6 in, 6 out]
  n378 = call "RSZVB Get Converter Source Frequency.vi"() -> ()  [unwired: 6 in, 6 out]
  n379 = call "RSZVB Get Local Oscilator B State.vi"() -> ()  [unwired: 9 in, 3 out]
  n380 = call "RSZVB Get Port Impedances Renormalization.vi"() -> ()  [unwired: 9 in, 3 out]
  n381 = call "RSZVB Get IF Gain Reference Channel.vi"() -> ()  [unwired: 9 in, 3 out]
  n382 = call "RSZVB Get Permanent Signal Generator State.vi"() -> ()  [unwired: 9 in, 3 out]
  n383 = call "RSZVB Get Source Combiner State.vi"() -> ()  [unwired: 9 in, 3 out]
  n384 = call "RSZVB Get TDIF State.vi"() -> ()  [unwired: 9 in, 3 out]
  n385 = call "RSZVB Set TDIF Amplitude Imbalance Stop Power.vi"() -> ()  [unwired: 10 in, 2 out]
  n386 = call "RSZVB Get TDIF Phase Imbalance Start Phase.vi"() -> ()  [unwired: 9 in, 3 out]
  n387 = call "RSZVB Set TDIF Compensation State.vi"() -> ()  [unwired: 10 in, 2 out]
  n388 = call "RSZVB Set Internal Combiner.vi"() -> ()  [unwired: 10 in, 2 out]
  n389 = call "RSZVB Set External Signal Generator Input.vi"() -> ()  [unwired: 10 in, 2 out]
  n390 = call "RSZVB Get TRM Measure Input.vi"() -> ()  [unwired: 9 in, 3 out]
  n391 = call "RSZVB Set TRM Pulse Modulator State.vi"() -> ()  [unwired: 10 in, 2 out]
  n392 = call "RSZVB Get TRM User Measurement Path Extension State.vi"() -> ()  [unwired: 9 in, 3 out]
  n393 = call "RSZVB Set TRM Pulse Generator Invert Source.vi"() -> ()  [unwired: 10 in, 2 out]
  n394 = call "RSZVB Get IMOD Lower Tone Source.vi"() -> ()  [unwired: 8 in, 4 out]
  n395 = call "RSZVB Get IMOD Enhanced Wave Correction.vi"() -> ()  [unwired: 9 in, 3 out]
  n396 = call "RSZVB Get Noise Figure Detector Measurement Time.vi"() -> ()  [unwired: 9 in, 3 out]
  n397 = call "RSZVB Get Noise Figure Narowband DUT.vi"() -> ()  [unwired: 9 in, 3 out]
  n398 = call "RSZVB Get Virtual Transform Balanced State.vi"() -> ()  [unwired: 9 in, 3 out]
  n399 = call "RSZVB Load And Interchange Balanced Port Circuit Model Data.vi"() -> ()  [unwired: 10 in, 2 out]
  n400 = call "RSZVB Get Virtual Transform Single Ended Circuit Model.vi"() -> ()  [unwired: 9 in, 3 out]
  n401 = call "RSZVB Get Virtual Transform Ground Loop.vi"() -> ()  [unwired: 9 in, 3 out]
  n402 = call "RSZVB Set Virtual Transform Port Pair.vi"() -> ()  [unwired: 14 in, 2 out]
  n403 = call "RSZVB Set Trace Math State.vi"() -> ()  [unwired: 10 in, 2 out]
  n404 = call "RSZVB Get Trace Transform Domain.vi"() -> ()  [unwired: 9 in, 3 out]
  n405 = call "RSZVB Set Display Line.vi"() -> ()  [unwired: 10 in, 2 out]
  n406 = call "RSZVB Set Stop Frequency.vi"() -> ()  [unwired: 10 in, 2 out]
  n407 = call "RSZVB Set Power.vi"() -> ()  [unwired: 10 in, 2 out]
  n408 = call "RSZVB Set Stop Power.vi"() -> ()  [unwired: 10 in, 2 out]
  n409 = call "RSZVB Get Receiver Step Attenuators.vi"() -> ()  [unwired: 9 in, 3 out]
  n410 = call "RSZVB Set Generator Attenuator Mode.vi"() -> ()  [unwired: 10 in, 2 out]
  n411 = call "RSZVB Set Meas Bandwidth Selectivity.vi"() -> ()  [unwired: 10 in, 2 out]
  n412 = call "RSZVB Set Average Factor.vi"() -> ()  [unwired: 10 in, 2 out]
  n413 = call "RSZVB Define Port Pair.vi"() -> ()  [unwired: 10 in, 2 out]
  n414 = call "RSZVB Set Converter Power Offset.vi"() -> ()  [unwired: 10 in, 2 out]
  n415 = call "RSZVB Set Type Of Port Transfer Model.vi"() -> ()  [unwired: 10 in, 2 out]
  n416 = call "RSZVB Set Converter User Data Set Directory.vi"() -> ()  [unwired: 10 in, 2 out]
  n417 = call "RSZVB Set Port Waveguide Attenuator.vi"() -> ()  [unwired: 10 in, 2 out]
  n418 = call "RSZVB Get Port Waveguide Attenuator Offset.vi"() -> ()  [unwired: 9 in, 3 out]
  n419 = call "RSZVB Set Simultaneous Measurement Of Ports Groups.vi"() -> ()  [unwired: 10 in, 2 out]
  n420 = call "RSZVB Set Simultaneous Measurement Minimum Frequency Offset Bandwidth Factor.vi"() -> ()  [unwired: 10 in, 2 out]
  n421 = call "RSZVB Get IMOD Max Order.vi"() -> ()  [unwired: 9 in, 3 out]
  n422 = call "RSZVB Start IMOD Receiver Power Calibration.vi"() -> ()  [unwired: 10 in, 2 out]
  n423 = call "RSZVB Define Noise Figure Calibration Settings.vi"() -> ()  [unwired: 10 in, 2 out]
  n424 = call "RSZVB Query Measurement Parameters.vi"() -> ()  [unwired: 9 in, 3 out]
  n425 = call "RSZVB Select PAE Measurement.vi"() -> ()  [unwired: 10 in, 2 out]
  n426 = call "RSZVB Window Close.vi"() -> ()  [unwired: 10 in, 2 out]
  n427 = call "RSZVB Print Setup.vi"() -> ()  [unwired: 18 in, 2 out]
  n428 = call "RSZVB File Catalog.vi"() -> ()  [unwired: 9 in, 3 out]
  n429 = call "RSZVB Write From File To Instrument.vi"() -> ()  [unwired: 10 in, 2 out]
  n430 = call "RSZVB Select More S-Parameters.vi"() -> ()  [unwired: 10 in, 2 out]
  n431 = call "RSZVB Select More Ratios.vi"() -> ()  [unwired: 14 in, 2 out]
  n432 = call "RSZVB Select More Wave Quantities.vi"() -> ()  [unwired: 10 in, 2 out]
  n433 = call "RSZVB Select More Impedances.vi"() -> ()  [unwired: 10 in, 2 out]
  n434 = call "RSZVB Select More Admitances.vi"() -> ()  [unwired: 10 in, 2 out]
  n435 = call "RSZVB Set Trace Unit.vi"() -> ()  [unwired: 10 in, 2 out]
  n436 = call "RSZVB Set Trace Bottom.vi"() -> ()  [unwired: 10 in, 2 out]
  n437 = call "RSZVB Set Trace Ref Value By Name.vi"() -> ()  [unwired: 10 in, 2 out]
  n438 = call "RSZVB Get Trace Top.vi"() -> ()  [unwired: 9 in, 3 out]
  n439 = call "RSZVB Set Time Domain Start Time.vi"() -> ()  [unwired: 10 in, 2 out]
  n440 = call "RSZVB Set Time Domain Center Time.vi"() -> ()  [unwired: 10 in, 2 out]
  n441 = call "RSZVB Set Time Domain Time Axis Scaling.vi"() -> ()  [unwired: 10 in, 2 out]
  n442 = call "RSZVB Set Time Domain Transformation Type.vi"() -> ()  [unwired: 10 in, 2 out]
  n443 = call "RSZVB Set Time Domain Transformation Sideband Suppression.vi"() -> ()  [unwired: 10 in, 2 out]
  n444 = call "RSZVB Get Time Gate State.vi"() -> ()  [unwired: 9 in, 3 out]
  n445 = call "RSZVB Get Trace Smoothing.vi"() -> ()  [unwired: 8 in, 4 out]
  n446 = call "RSZVB Set Marker Target Value.vi"() -> ()  [unwired: 10 in, 2 out]
  n447 = call "RSZVB Marker Bandstop Search.vi"() -> ()  [unwired: 10 in, 2 out]
  n448 = call "RSZVB Set Center To Marker.vi"() -> ()  [unwired: 10 in, 2 out]
  n449 = call "RSZVB Get Limit Check.vi"() -> ()  [unwired: 9 in, 3 out]
  n450 = call "RSZVB Edit Limit Line Segment.vi"() -> ()  [unwired: 14 in, 2 out]
  n451 = call "RSZVB Recall Limit Line.vi"() -> ()  [unwired: 10 in, 2 out]
  n452 = call "RSZVB Get Partial Measurement Resolution Bandwidth Mode.vi"() -> ()  [unwired: 9 in, 3 out]
  n453 = call "RSZVB Get Channel Bits.vi"() -> ()  [unwired: 9 in, 3 out]
  n454 = call "RSZVB Get UI Data.vi"() -> ()  [unwired: 9 in, 3 out]
  n455 = call "RSZVB Get UI Port Binary Data.vi"() -> ()  [unwired: 9 in, 3 out]
  n456 = call "RSZVB Get Reference Frequency.vi"() -> ()  [unwired: 9 in, 3 out]
  n457 = call "RSZVB Get Pulse Generator State.vi"() -> ()  [unwired: 9 in, 3 out]
  n458 = call "RSZVB Configure Pulse Generators.vi"() -> ()  [unwired: 10 in, 2 out]
  n459 = call "RSZVB Diagram Area Title.vi"() -> ()  [unwired: 10 in, 2 out]
  n460 = call "RSZVB Load Color Scheme.vi"() -> ()  [unwired: 10 in, 2 out]
  n461 = call "RSZVB Get Channel Info.vi"() -> ()  [unwired: 9 in, 3 out]
  n462 = call "RSZVB Get Trace Color State.vi"() -> ()  [unwired: 9 in, 3 out]
  n463 = call "RSZVB Get Power Port Limit Value.vi"() -> ()  [unwired: 9 in, 3 out]
  n464 = call "RSZVB Get Preset Settings State.vi"() -> ()  [unwired: 9 in, 3 out]
  n465 = call "RSZVB Get User Defined Preset File.vi"() -> ()  [unwired: 9 in, 3 out]
  n466 = call "RSZVB Query Frequency Range.vi"() -> ()  [unwired: 8 in, 4 out]
  n467 = call "RSZVB Query External Generator Count.vi"() -> ()  [unwired: 9 in, 3 out]
  n468 = call "RSZVB Query External Power Meter Numbers.vi"() -> ()  [unwired: 9 in, 3 out]
  n469 = call "RSZVB Get Alarm Sounds State.vi"() -> ()  [unwired: 9 in, 3 out]
  n470 = call "RSZVB Get Data Transfer.vi"() -> ()  [unwired: 9 in, 3 out]
  n471 = call "RSZVB Get Frequency Conversion Source.vi"() -> ()  [unwired: 9 in, 3 out]
  n472 = call "RSZVB Get Power Coeficients Default.vi"() -> ()  [unwired: 9 in, 3 out]
  n473 = call "RSZVB Generate System Report.vi"() -> ()  [unwired: 10 in, 2 out]
  n474 = call "RSZVB Get Remote Display Title.vi"() -> ()  [unwired: 9 in, 3 out]
  n475 = call "RSZVB Configure Calibration Standard.vi"() -> ()  [unwired: 26 in, 2 out]
  n476 = call "RSZVB Get Source Power Calibration State.vi"() -> ()  [unwired: 9 in, 3 out]
  n477 = call "RSZVB Get B Wave Receiver Power Calibration State.vi"() -> ()  [unwired: 9 in, 3 out]
  n478 = call "RSZVB Get Electrical Length.vi"() -> ()  [unwired: 9 in, 3 out]
  n479 = call "RSZVB Set Permittivity.vi"() -> ()  [unwired: 10 in, 2 out]
  n480 = call "RSZVB Set Loss At Frequency.vi"() -> ()  [unwired: 10 in, 2 out]
  n481 = call "RSZVB Auto Length.vi"() -> ()  [unwired: 10 in, 2 out]
  n482 = call "RSZVB Save Fixture Compensation Data.vi"() -> ()  [unwired: 10 in, 2 out]
  n483 = call "RSZVB Write Source Power Correction Data.vi"() -> ()  [unwired: 10 in, 2 out]
  n484 = call "RSZVB Get Source Power Calibration Paramater Wave.vi"() -> ()  [unwired: 9 in, 3 out]
  n485 = call "RSZVB Get Source Power Calibration Converter State.vi"() -> ()  [unwired: 9 in, 3 out]
  n486 = call "RSZVB Set A Wave Receiver Power Calibration State.vi"() -> ()  [unwired: 10 in, 2 out]
  n487 = call "RSZVB Set Power Sensor Position.vi"() -> ()  [unwired: 10 in, 2 out]
  n488 = call "RSZVB Get Loss List Number of Values.vi"() -> ()  [unwired: 9 in, 3 out]
  n489 = call "RSZVB Delete Power Loss List Single Point.vi"() -> ()  [unwired: 10 in, 2 out]
  n490 = call "RSZVB Set Receiver Power Correction State.vi"() -> ()  [unwired: 10 in, 2 out]
  n491 = call "RSZVB Get Calibration Data Ports.vi"() -> ()  [unwired: 9 in, 3 out]
  n492 = call "RSZVB Get Automatic Power Reduction State.vi"() -> ()  [unwired: 9 in, 3 out]
  n493 = call "RSZVB Get Enhanced Wave Correction.vi"() -> ()  [unwired: 9 in, 3 out]
  n494 = call "RSZVB Set Calibration Kit With Label.vi"() -> ()  [unwired: 10 in, 2 out]
  n495 = call "RSZVB Rename Calibration Kit.vi"() -> ()  [unwired: 10 in, 2 out]
  n496 = call "RSZVB Calibration Connector Catalog.vi"() -> ()  [unwired: 9 in, 3 out]
  n497 = call "RSZVB Get Calibrations Number.vi"() -> ()  [unwired: 9 in, 3 out]
  n498 = call "RSZVB Get Source Power Calibration Port State.vi"() -> ()  [unwired: 9 in, 3 out]
  n499 = call "RSZVB Get Verification Sweep State.vi"() -> ()  [unwired: 9 in, 3 out]
  n500 = call "RSZVB Calibration Auto Type Simplified.vi"() -> ()  [unwired: 14 in, 2 out]
  n501 = call "RSZVB Get Calibration Auto Assignment Definition.vi"() -> ()  [unwired: 6 in, 10 out]
  n502 = call "RSZVB Set Calibration Data Default State.vi"() -> ()  [unwired: 10 in, 2 out]
  n503 = call "RSZVB Set Same Connector Type at All Ports.vi"() -> ()  [unwired: 10 in, 2 out]
  n504 = call "RSZVB Set Same Sweep Setup.vi"() -> ()  [unwired: 10 in, 2 out]
  n505 = call "RSZVB Initiate Source Power Calibration.vi"() -> ()  [unwired: 10 in, 2 out]
  n506 = call "RSZVB Channel Delete.vi"() -> ()  [unwired: 10 in, 2 out]
  n507 = call "RSZVB Channel Get Active.vi"() -> ()  [unwired: 9 in, 3 out]
  n508 = call "RSZVB Read Calibration Data.vi"() -> ()  [unwired: 9 in, 3 out]
  n509 = call "RSZVB Start Calibration.vi"() -> ()  [unwired: 10 in, 2 out]
  n510 = call "RSZVB Get Calibration Reference Plane Shift Specific.vi"() -> ()  [unwired: 9 in, 3 out]
  n511 = call "RSZVB Set Check Ripple Limit Range Segment.vi"() -> ()  [unwired: 10 in, 2 out]
  n512 = call "RSZVB Set Ripple Fail Beep On.vi"() -> ()  [unwired: 10 in, 2 out]
  n513 = call "RSZVB Delete All Ripple Limit Ranges.vi"() -> ()  [unwired: 10 in, 2 out]
  n514 = call "RSZVB Save Recall Ripple Limit.vi"() -> ()  [unwired: 10 in, 2 out]
  n515 = call "RSZVB Set Marker Search Range Show.vi"() -> ()  [unwired: 10 in, 2 out]
  n516 = call "RSZVB Get Sweep Segment Frequency Span.vi"() -> ()  [unwired: 9 in, 3 out]
  n517 = call "RSZVB Set PI Controller Gain.vi"() -> ()  [unwired: 10 in, 2 out]
  n518 = call "RSZVB Modify Source Power Calibration Settings.vi"() -> ()  [unwired: 18 in, 2 out]
  n519 = call "RSZVB Redefine Segment.vi"() -> ()  [unwired: 18 in, 2 out]
  n520 = call "RSZVB Get Sweep Segment State.vi"() -> ()  [unwired: 9 in, 3 out]
  n521 = call "RSZVB Get Sweep Segment Number Of Points.vi"() -> ()  [unwired: 9 in, 3 out]
  n522 = call "RSZVB Get Sweep Segment Independent Power.vi"() -> ()  [unwired: 9 in, 3 out]
  n523 = call "RSZVB Get Sweep Segment Spur Avoid.vi"() -> ()  [unwired: 9 in, 3 out]
  n524 = call "RSZVB Get Sweep Segment Independent Selectivity.vi"() -> ()  [unwired: 9 in, 3 out]
  n525 = call "RSZVB Get Sweep Segment Point Delay.vi"() -> ()  [unwired: 9 in, 3 out]
  n526 = call "RSZVB Get Sweep Selective Segment Triggering.vi"() -> ()  [unwired: 9 in, 3 out]
  n527 = call "RSZVB Set Display Results State.vi"() -> ()  [unwired: 10 in, 2 out]
  n528 = call "RSZVB Get Renormalization Impedance.vi"() -> ()  [unwired: 9 in, 3 out]
  n529 = call "RSZVB Get Pulse Time Start.vi"() -> ()  [unwired: 9 in, 3 out]
  n530 = call "RSZVB Get Pulse Coupled Section Limit Lines State.vi"() -> ()  [unwired: 9 in, 3 out]
  n531 = call "RSZVB Get Pulse Evaluation Section Stop.vi"() -> ()  [unwired: 9 in, 3 out]
  n532 = call "RSZVB Get Renormalization State.vi"() -> ()  [unwired: 9 in, 3 out]
  n533 = call "RSZVB Get Number Of Stages.vi"() -> ()  [unwired: 9 in, 3 out]
  n534 = call "RSZVB Get RF Signal Port.vi"() -> ()  [unwired: 9 in, 3 out]
  n535 = call "RSZVB Get External Power Meter.vi"() -> ()  [unwired: 9 in, 3 out]
  n536 = call "RSZVB Get Mixer Delay Measurement Setup.vi"() -> ()  [unwired: 9 in, 3 out]
  n537 = call "RSZVB Start Mixer Delay Calibration Sweep.vi"() -> ()  [unwired: 10 in, 2 out]
  n538 = call "RSZVB Set Mixer Delay Combiner State.vi"() -> ()  [unwired: 10 in, 2 out]
  n539 = call "RSZVB Get Mixer Constant Delay Enabled.vi"() -> ()  [unwired: 9 in, 3 out]
  n540 = call "RSZVB Get Vector Mixer Mode.vi"() -> ()  [unwired: 9 in, 3 out]
  n541 = call "RSZVB Set AUX Mixer Port.vi"() -> ()  [unwired: 10 in, 2 out]
  n542 = call "RSZVB Get Trace Display State.vi"() -> ()  [unwired: 9 in, 3 out]
  n543 = call "RSZVB Trace Unassign Diagram Area.vi"() -> ()  [unwired: 10 in, 2 out]
  n544 = call "RSZVB Channel Trace Rename.vi"() -> ()  [unwired: 10 in, 2 out]
  n545 = call "RSZVB Trace Get Channel Number.vi"() -> ()  [unwired: 9 in, 3 out]
  n546 = call "RSZVB Set Trace Evaluation Range Show.vi"() -> ()  [unwired: 10 in, 2 out]
  n547 = call "RSZVB Set Pulse Generator Delay.vi"() -> ()  [unwired: 10 in, 2 out]
  n548 = call "RSZVB Get Harmonic Measurement State.vi"() -> ()  [unwired: 9 in, 3 out]
  n549 = call "RSZVB Set Harmonic Receive Port.vi"() -> ()  [unwired: 10 in, 2 out]
  n550 = call "RSZVB Load Mixer Delay Values.vi"() -> ()  [unwired: 10 in, 2 out]
  n551 = call "RSZVB Get Trigger Source.vi"() -> ()  [unwired: 9 in, 3 out]
  n552 = call "RSZVB Set Generator Port Trigger Delay.vi"() -> ()  [unwired: 10 in, 2 out]
  n553 = call "RSZVB Get Triggered Meas Sequence.vi"() -> ()  [unwired: 9 in, 3 out]
  n554 = call "RSZVB Delete Port Pair.vi"() -> ()  [unwired: 10 in, 2 out]
  n555 = call "RSZVB Get Pulse Generator Type.vi"() -> ()  [unwired: 9 in, 3 out]
  n556 = call "RSZVB Get Pulse Generator Polarity.vi"() -> ()  [unwired: 9 in, 3 out]
  n557 = call "RSZVB Set Pulse Train Segment Start.vi"() -> ()  [unwired: 10 in, 2 out]
  n558 = call "RSZVB Get Internal Combiner.vi"() -> ()  [unwired: 9 in, 3 out]
  n559 = call "RSZVB Get External Signal Generator Input.vi"() -> ()  [unwired: 9 in, 3 out]
  n560 = call "RSZVB Configure Frequency Settings.vi"() -> ()  [unwired: 10 in, 2 out]
  n561 = call "RSZVB Set Coherent Signal Amplitude.vi"() -> ()  [unwired: 10 in, 2 out]
  n562 = call "RSZVB Set Spurious Avoidance.vi"() -> ()  [unwired: 10 in, 2 out]
  n563 = call "RSZVB Set ALC Port State.vi"() -> ()  [unwired: 10 in, 2 out]
  n564 = call "RSZVB Set ALC Port Bandwidth.vi"() -> ()  [unwired: 10 in, 2 out]
  n565 = call "RSZVB Set ALC Low Phase Noise Mode.vi"() -> ()  [unwired: 10 in, 2 out]
  n566 = call "RSZVB Set ALC Port Start Offset.vi"() -> ()  [unwired: 10 in, 2 out]
  n567 = call "RSZVB Configure Port PI Controller.vi"() -> ()  [unwired: 10 in, 2 out]
  n568 = call "RSZVB Get SAW State.vi"() -> ()  [unwired: 9 in, 3 out]
  n569 = call "RSZVB Set SAW Simulation Type.vi"() -> ()  [unwired: 10 in, 2 out]
  n570 = call "RSZVB Trace Export Data With Options.vi"() -> ()  [unwired: 10 in, 2 out]
  n571 = call "RSZVB Trace Export Data Ports.vi"() -> ()  [unwired: 14 in, 2 out]
  n572 = call "RSZVB Set Linearity Deviation State.vi"() -> ()  [unwired: 10 in, 2 out]
  n573 = call "RSZVB Get Linearity Deviation Slope.vi"() -> ()  [unwired: 9 in, 3 out]
  n574 = call "RSZVB Get Sweep Time.vi"() -> ()  [unwired: 9 in, 3 out]
  n575 = call "RSZVB Get Simultaneous Measurement Of Ports Groups.vi"() -> ()  [unwired: 9 in, 3 out]
  n576 = call "RSZVB Get Simultaneous Measurement Minimum Frequency Offset Bandwidth Factor.vi"() -> ()  [unwired: 9 in, 3 out]
  n577 = call "RSZVB Get Frequency Stimulus.vi"() -> ()  [unwired: 9 in, 3 out]
  n578 = call "RSZVB Configure Power Settings.vi"() -> ()  [unwired: 10 in, 2 out]
  n579 = call "RSZVB Set Noise Figure RF Image Correction.vi"() -> ()  [unwired: 10 in, 2 out]
  n580 = call "RSZVB Delete Memory Trace.vi"() -> ()  [unwired: 10 in, 2 out]
  n581 = call "RSZVB Trace Response Data All.vi"() -> ()  [unwired: 9 in, 3 out]
  n582 = call "RSZVB Trace Response Single Sweep Data Forward.vi"() -> ()  [unwired: 9 in, 3 out]
  n583 = call "RSZVB Trace Response Data ZVR.vi"() -> ()  [unwired: 9 in, 3 out]
  n584 = call "RSZVB Set Generator Step Attenuators.vi"() -> ()  [unwired: 10 in, 2 out]
  n585 = call "RSZVB Get Generator Attenuator Mode.vi"() -> ()  [unwired: 9 in, 3 out]
  n586 = call "RSZVB Get Meas Bandwidth Selectivity.vi"() -> ()  [unwired: 9 in, 3 out]
  n587 = call "RSZVB Get Average Factor.vi"() -> ()  [unwired: 9 in, 3 out]
  n588 = call "RSZVB Set Frequency Step Size.vi"() -> ()  [unwired: 10 in, 2 out]
  n589 = call "RSZVB Set Power Meter Frequency Conversion.vi"() -> ()  [unwired: 10 in, 2 out]
  n590 = call "RSZVB Set Measure A Waves State.vi"() -> ()  [unwired: 10 in, 2 out]
  n591 = call "RSZVB Set Logical Port Common Ref Impedance.vi"() -> ()  [unwired: 10 in, 2 out]
  n592 = call "RSZVB Set Physical Port Ref Impedance.vi"() -> ()  [unwired: 10 in, 2 out]
  n593 = call "RSZVB Set RF Signal Source State.vi"() -> ()  [unwired: 10 in, 2 out]
  n594 = call "RSZVB Set Port Power Generator Offset.vi"() -> ()  [unwired: 10 in, 2 out]
  n595 = call "RSZVB Set TDIF Amplitude Imbalance Logical Port.vi"() -> ()  [unwired: 10 in, 2 out]
  n596 = call "RSZVB Get TDIF Amplitude Imbalance Stop Power.vi"() -> ()  [unwired: 9 in, 3 out]
  n597 = call "RSZVB Set TDIF Phase Imbalance Stop Phase.vi"() -> ()  [unwired: 10 in, 2 out]
  n598 = call "RSZVB Get TDIF Compensation State.vi"() -> ()  [unwired: 9 in, 3 out]
  n599 = call "RSZVB Set IMOD Upper Tone Source.vi"() -> ()  [unwired: 10 in, 2 out]
  n600 = call "RSZVB Set IMOD Measurement Order.vi"() -> ()  [unwired: 10 in, 2 out]
  n601 = call "RSZVB Set Noise Figure Measurement Mode.vi"() -> ()  [unwired: 10 in, 2 out]
  n602 = call "RSZVB Set Time Gate Stop Time.vi"() -> ()  [unwired: 10 in, 2 out]
  n603 = call "RSZVB Get Time Gate Type.vi"() -> ()  [unwired: 9 in, 3 out]
  n604 = call "RSZVB Set Time Gate Shape.vi"() -> ()  [unwired: 10 in, 2 out]
  n605 = call "RSZVB Get Time Gate Display State.vi"() -> ()  [unwired: 9 in, 3 out]
  n606 = call "RSZVB Configure Trigger Periodic.vi"() -> ()  [unwired: 10 in, 2 out]
  n607 = call "RSZVB Get Default Configuration State.vi"() -> ()  [unwired: 9 in, 3 out]
  n608 = call "RSZVB Get Converter Power Offset.vi"() -> ()  [unwired: 8 in, 4 out]
  n609 = call "RSZVB Get Type Of Port Transfer Model.vi"() -> ()  [unwired: 9 in, 3 out]
  n610 = call "RSZVB Get Converter User Data Set Directory.vi"() -> ()  [unwired: 9 in, 3 out]
  n611 = call "RSZVB Get Port Waveguide Attenuator Type.vi"() -> ()  [unwired: 9 in, 3 out]
  n612 = call "RSZVB Set Port Electronic Power Treshold.vi"() -> ()  [unwired: 10 in, 2 out]
  n613 = call "RSZVB Set IMOD Two Tone Output.vi"() -> ()  [unwired: 10 in, 2 out]
  n614 = call "RSZVB Set IMOD Distortion Measurement Calibration State.vi"() -> ()  [unwired: 10 in, 2 out]
  n615 = call "RSZVB Start Noise Figure Calibration.vi"() -> ()  [unwired: 10 in, 2 out]
  n616 = call "RSZVB Set Virtual Transform Balanced Port.vi"() -> ()  [unwired: 14 in, 2 out]
  n617 = call "RSZVB Set Virtual Transform Single Ended State.vi"() -> ()  [unwired: 10 in, 2 out]
  n618 = call "RSZVB Load Single Ended Port Circuit Model Data.vi"() -> ()  [unwired: 10 in, 2 out]
  n619 = call "RSZVB Set Virtual Transform Ground Loop Circuit Model.vi"() -> ()  [unwired: 10 in, 2 out]
  n620 = call "RSZVB Get Virtual Transform Port Pair.vi"() -> ()  [unwired: 13 in, 3 out]
  n621 = call "RSZVB Get Marker Stimulus.vi"() -> ()  [unwired: 9 in, 3 out]
  n622 = call "RSZVB Get Reference Marker Stimulus.vi"() -> ()  [unwired: 9 in, 3 out]
  n623 = call "RSZVB Get Reference Fixed Marker.vi"() -> ()  [unwired: 9 in, 3 out]
  n624 = call "RSZVB Set Discrete Marker.vi"() -> ()  [unwired: 10 in, 2 out]
  n625 = call "RSZVB Get Marker Format.vi"() -> ()  [unwired: 9 in, 3 out]
  n626 = call "RSZVB Marker x dB Bandwidth ZVR.vi"() -> ()  [unwired: 10 in, 2 out]
  n627 = call "RSZVB Set Limit Line Fail Beep.vi"() -> ()  [unwired: 10 in, 2 out]
  n628 = call "RSZVB Read Limit Line Segment List.vi"() -> ()  [unwired: 8 in, 8 out]
  n629 = call "RSZVB Recall Limit Line With Options.vi"() -> ()  [unwired: 10 in, 2 out]
  n630 = call "RSZVB Get Display Line.vi"() -> ()  [unwired: 8 in, 4 out]
  n631 = call "RSZVB Get Stop Frequency.vi"() -> ()  [unwired: 9 in, 3 out]
  n632 = call "RSZVB Get Power.vi"() -> ()  [unwired: 9 in, 3 out]
  n633 = call "RSZVB Get Stop Power.vi"() -> ()  [unwired: 9 in, 3 out]
  n634 = call "RSZVB Set Generator Port Resolution Bandwidth.vi"() -> ()  [unwired: 10 in, 2 out]
  n635 = call "RSZVB Send Channel Trigger.vi"() -> ()  [unwired: 10 in, 2 out]
  n636 = call "RSZVB Get Sweep Single.vi"() -> ()  [unwired: 9 in, 3 out]
  n637 = call "RSZVB Get Group Of Measured Ports.vi"() -> ()  [unwired: 8 in, 4 out]
  n638 = call "RSZVB Get Balanced Port.vi"() -> ()  [unwired: 8 in, 4 out]
  n639 = call "RSZVB Set Differential Mode Impedance.vi"() -> ()  [unwired: 10 in, 2 out]
  n640 = call "RSZVB Set TRM Combiner State.vi"() -> ()  [unwired: 10 in, 2 out]
  n641 = call "RSZVB Get TRM Pulse Modulator State.vi"() -> ()  [unwired: 9 in, 3 out]
  n642 = call "RSZVB Set TRM Pulse Modulator Source.vi"() -> ()  [unwired: 10 in, 2 out]
  n643 = call "RSZVB Get TRM Pulse Generator Invert Source.vi"() -> ()  [unwired: 9 in, 3 out]
  n644 = call "RSZVB Select More Ratios With Detector.vi"() -> ()  [unwired: 14 in, 2 out]
  n645 = call "RSZVB Select More Wave Quantities With Detector.vi"() -> ()  [unwired: 14 in, 2 out]
  n646 = call "RSZVB Get Trace Math State.vi"() -> ()  [unwired: 9 in, 3 out]
  n647 = call "RSZVB Set Trace Transform Conversion.vi"() -> ()  [unwired: 10 in, 2 out]
  n648 = call "RSZVB Window List.vi"() -> ()  [unwired: 9 in, 3 out]
  n649 = call "RSZVB Setup Save.vi"() -> ()  [unwired: 10 in, 2 out]
  n650 = call "RSZVB Define PAE Measurement.vi"() -> ()  [unwired: 10 in, 2 out]
  n651 = call "RSZVB Get Trace Unit.vi"() -> ()  [unwired: 9 in, 3 out]
  n652 = call "RSZVB Get Trace Bottom.vi"() -> ()  [unwired: 9 in, 3 out]
  n653 = call "RSZVB Get Trace Ref Value.vi"() -> ()  [unwired: 9 in, 3 out]
  n654 = call "RSZVB Get Time Domain Start Time.vi"() -> ()  [unwired: 9 in, 3 out]
  n655 = call "RSZVB Get Time Domain Center Time.vi"() -> ()  [unwired: 9 in, 3 out]
  n656 = call "RSZVB Get Time Domain Time Axis Scaling.vi"() -> ()  [unwired: 9 in, 3 out]
  n657 = call "RSZVB Get Time Domain Transformation Type.vi"() -> ()  [unwired: 9 in, 3 out]
  n658 = call "RSZVB Get Time Domain Transformation Sideband Suppression.vi"() -> ()  [unwired: 9 in, 3 out]
  n659 = call "RSZVB Set Harmonic Grid and Keep.vi"() -> ()  [unwired: 10 in, 2 out]
  n660 = call "RSZVB Set Continuous Extrapolation.vi"() -> ()  [unwired: 10 in, 2 out]
  n661 = call "RSZVB Get Marker Target Value.vi"() -> ()  [unwired: 9 in, 3 out]
  n662 = call "RSZVB Set Marker Search Mode.vi"() -> ()  [unwired: 10 in, 2 out]
  n663 = call "RSZVB Set UI Signal Pin 20.vi"() -> ()  [unwired: 10 in, 2 out]
  n664 = call "RSZVB Set UI Port Next State.vi"() -> ()  [unwired: 10 in, 2 out]
  n665 = call "RSZVB Define Pulse Generator.vi"() -> ()  [unwired: 14 in, 2 out]
  n666 = call "RSZVB Configure Calibration Standard With Label.vi"() -> ()  [unwired: 10 in, 2 out]
  n667 = call "RSZVB Diagram Area Name.vi"() -> ()  [unwired: 10 in, 2 out]
  n668 = call "RSZVB Set Frequency Info.vi"() -> ()  [unwired: 10 in, 2 out]
  n669 = call "RSZVB Set Marker Color State.vi"() -> ()  [unwired: 10 in, 2 out]
  n670 = call "RSZVB Trace Set RGB Color.vi"() -> ()  [unwired: 14 in, 2 out]
  n671 = call "RSZVB Set Analyzer Hostname.vi"() -> ()  [unwired: 10 in, 2 out]
  n672 = call "RSZVB Set Power Port Limit Direct Generator And Receiver State.vi"() -> ()  [unwired: 10 in, 2 out]
  n673 = call "RSZVB System Keylock.vi"() -> ()  [unwired: 10 in, 2 out]
  n674 = call "RSZVB Query External Generator Numbers.vi"() -> ()  [unwired: 9 in, 3 out]
  n675 = call "RSZVB Auto Zeroing External Power Meter.vi"() -> ()  [unwired: 10 in, 2 out]
  n676 = call "RSZVB Set Restart Behavior.vi"() -> ()  [unwired: 10 in, 2 out]
  n677 = call "RSZVB Set Error Display State.vi"() -> ()  [unwired: 10 in, 2 out]
  n678 = call "RSZVB Set Fast Multiport Correction.vi"() -> ()  [unwired: 10 in, 2 out]
  n679 = call "RSZVB Query Extension Unit Device ID.vi"() -> ()  [unwired: 9 in, 3 out]
  n680 = call "RSZVB Set Calculation of Bandfilter Center Frequency.vi"() -> ()  [unwired: 10 in, 2 out]
  n681 = call "RSZVB Get Calibration Data Throughs.vi"() -> ()  [unwired: 9 in, 3 out]
  n682 = call "RSZVB Get All Calibration Units.vi"() -> ()  [unwired: 9 in, 3 out]
  n683 = call "RSZVB Set Load Matching Correction.vi"() -> ()  [unwired: 10 in, 2 out]
  n684 = call "RSZVB Set Calibration Kit User Connector Type.vi"() -> ()  [unwired: 10 in, 2 out]
  n685 = call "RSZVB Get Calibration Kit Label.vi"() -> ()  [unwired: 9 in, 3 out]
  n686 = call "RSZVB Configure Mechanical Length.vi"() -> ()  [unwired: 10 in, 2 out]
  n687 = call "RSZVB Get Permittivity.vi"() -> ()  [unwired: 9 in, 3 out]
  n688 = call "RSZVB Get Loss At Frequency.vi"() -> ()  [unwired: 9 in, 3 out]
  n689 = call "RSZVB Auto Length And Loss.vi"() -> ()  [unwired: 10 in, 2 out]
  n690 = call "RSZVB Set Fixture Compensation Auto Length And Loss Calculation.vi"() -> ()  [unwired: 10 in, 2 out]
  n691 = call "RSZVB Get Source Power Calibration Paramater Start.vi"() -> ()  [unwired: 9 in, 3 out]
  n692 = call "RSZVB Read Receiver Power Correction Data.vi"() -> ()  [unwired: 8 in, 4 out]
  n693 = call "RSZVB Get Source Power Calibration Number Of Waves.vi"() -> ()  [unwired: 9 in, 3 out]
  n694 = call "RSZVB Set Source Power Calibration Convergence Factor.vi"() -> ()  [unwired: 10 in, 2 out]
  n695 = call "RSZVB Get A Wave Receiver Power Calibration State.vi"() -> ()  [unwired: 9 in, 3 out]
  n696 = call "RSZVB Get Power Sensor Position.vi"() -> ()  [unwired: 9 in, 3 out]
  n697 = call "RSZVB Set Power Loss List Coefficient.vi"() -> ()  [unwired: 10 in, 2 out]
  n698 = call "RSZVB Set Power Loss List Trace.vi"() -> ()  [unwired: 10 in, 2 out]
  n699 = call "RSZVB Get Receiver Power Correction State.vi"() -> ()  [unwired: 9 in, 3 out]
  n700 = call "RSZVB Calibration Retain Port Groups.vi"() -> ()  [unwired: 10 in, 2 out]
  n701 = call "RSZVB Get Calibration Data Parameters More Calibrations.vi"() -> ()  [unwired: 9 in, 7 out]
  n702 = call "RSZVB Set Reference Receiver Calibration State.vi"() -> ()  [unwired: 10 in, 2 out]
  n703 = call "RSZVB Initiate Calibration Auto Assignment.vi"() -> ()  [unwired: 10 in, 2 out]
  n704 = call "RSZVB Get Calibration Data Default State.vi"() -> ()  [unwired: 9 in, 3 out]
  n705 = call "RSZVB Delete Calibration Connector.vi"() -> ()  [unwired: 10 in, 2 out]
  n706 = call "RSZVB Get Same Connector Type at All Ports.vi"() -> ()  [unwired: 9 in, 3 out]
  n707 = call "RSZVB Get Same Sweep Setup.vi"() -> ()  [unwired: 9 in, 3 out]
  n708 = call "RSZVB Set Dummy Source Power Calibration State.vi"() -> ()  [unwired: 10 in, 2 out]
  n709 = call "RSZVB Set Source Power Calibration Generator State.vi"() -> ()  [unwired: 10 in, 2 out]
  n710 = call "RSZVB Get Check Ripple Limit Range Segment.vi"() -> ()  [unwired: 9 in, 3 out]
  n711 = call "RSZVB Get Ripple Fail Beep On.vi"() -> ()  [unwired: 9 in, 3 out]
  n712 = call "RSZVB Set Ripple Limit Physical Units.vi"() -> ()  [unwired: 10 in, 2 out]
  n713 = call "RSZVB Channel List.vi"() -> ()  [unwired: 9 in, 3 out]
  n714 = call "RSZVB Channel Rename.vi"() -> ()  [unwired: 10 in, 2 out]
  n715 = call "RSZVB Query Verification Sweep Results.vi"() -> ()  [unwired: 8 in, 4 out]
  n716 = call "RSZVB Get Marker Search Range Show.vi"() -> ()  [unwired: 9 in, 3 out]
  n717 = call "RSZVB Set Number Of Readings.vi"() -> ()  [unwired: 10 in, 2 out]
  n718 = call "RSZVB Set Other Sources State.vi"() -> ()  [unwired: 10 in, 2 out]
  n719 = call "RSZVB Set Calibration Power Offset.vi"() -> ()  [unwired: 10 in, 2 out]
  n720 = call "RSZVB Set Reference Receiver After First Cal Sweep.vi"() -> ()  [unwired: 10 in, 2 out]
  n721 = call "RSZVB Set Calibration Power Meter Readings.vi"() -> ()  [unwired: 10 in, 2 out]
  n722 = call "RSZVB Get PI Controller Gain.vi"() -> ()  [unwired: 9 in, 3 out]
  n723 = call "RSZVB Start Calibration Line.vi"() -> ()  [unwired: 10 in, 2 out]
  n724 = call "RSZVB Query Calibration Reference Plane Shift.vi"() -> ()  [unwired: 9 in, 3 out]
  n725 = call "RSZVB Write Calibration Data.vi"() -> ()  [unwired: 10 in, 2 out]
  n726 = call "RSZVB Set Internal Signal Source.vi"() -> ()  [unwired: 10 in, 2 out]
  n727 = call "RSZVB Get Trace Evaluation Range Show.vi"() -> ()  [unwired: 9 in, 3 out]
  n728 = call "RSZVB Get Display Results State.vi"() -> ()  [unwired: 9 in, 3 out]
  n729 = call "RSZVB Set Renormalization Mode.vi"() -> ()  [unwired: 10 in, 2 out]
  n730 = call "RSZVB Save Segment.vi"() -> ()  [unwired: 10 in, 2 out]
  n731 = call "RSZVB Set Harmonic Order.vi"() -> ()  [unwired: 10 in, 2 out]
  n732 = call "RSZVB Get Harmonic Receive Port.vi"() -> ()  [unwired: 9 in, 3 out]
  n733 = call "RSZVB Add New Segment.vi"() -> ()  [unwired: 10 in, 2 out]
  n734 = call "RSZVB Set Sweep Segment Start Frequency.vi"() -> ()  [unwired: 10 in, 2 out]
  n735 = call "RSZVB Set Sweep Segment Name.vi"() -> ()  [unwired: 10 in, 2 out]
  n736 = call "RSZVB Set Sweep Segment Meas Bandwidth.vi"() -> ()  [unwired: 10 in, 2 out]
  n737 = call "RSZVB Set Sweep Segment Independent Spur Avoid.vi"() -> ()  [unwired: 10 in, 2 out]
  n738 = call "RSZVB Set Sweep Segment Sweep Time.vi"() -> ()  [unwired: 10 in, 2 out]
  n739 = call "RSZVB Set Sweep Segment Independent Point Delay.vi"() -> ()  [unwired: 10 in, 2 out]
  n740 = call "RSZVB Set Sweep Segment Bits State.vi"() -> ()  [unwired: 10 in, 2 out]
  n741 = call "RSZVB Set Signal Source.vi"() -> ()  [unwired: 10 in, 2 out]
  n742 = call "RSZVB RF Source Calibration.vi"() -> ()  [unwired: 10 in, 2 out]
  n743 = call "RSZVB Set Mixer Delay LAN Connection.vi"() -> ()  [unwired: 10 in, 2 out]
  n744 = call "RSZVB Set Mixer Delay Aperture.vi"() -> ()  [unwired: 10 in, 2 out]
  n745 = call "RSZVB Get Mixer Delay Combiner State.vi"() -> ()  [unwired: 9 in, 3 out]
  n746 = call "RSZVB Set Mixer Delay Correction.vi"() -> ()  [unwired: 10 in, 2 out]
  n747 = call "RSZVB Load Mixer Delay Calibration Data.vi"() -> ()  [unwired: 10 in, 2 out]
  n748 = call "RSZVB Set Internal Signal Source AUX.vi"() -> ()  [unwired: 10 in, 2 out]
  n749 = call "RSZVB Get AUX Mixer Port.vi"() -> ()  [unwired: 9 in, 3 out]
  n750 = call "RSZVB Get Spurious Avoidance.vi"() -> ()  [unwired: 9 in, 3 out]
  n751 = call "RSZVB Get ALC Port State.vi"() -> ()  [unwired: 9 in, 3 out]
  n752 = call "RSZVB Get ALC Port Bandwidth.vi"() -> ()  [unwired: 9 in, 3 out]
  n753 = call "RSZVB Get ALC Low Phase Noise Mode.vi"() -> ()  [unwired: 9 in, 3 out]
  n754 = call "RSZVB Get ALC Port Start Offset.vi"() -> ()  [unwired: 9 in, 3 out]
  n755 = call "RSZVB Set Pulse Time Stop.vi"() -> ()  [unwired: 10 in, 2 out]
  n756 = call "RSZVB Set Pulse Evaluation Mode.vi"() -> ()  [unwired: 10 in, 2 out]
  n757 = call "RSZVB Set Pulse Section Limit Lines State.vi"() -> ()  [unwired: 10 in, 2 out]
  n758 = call "RSZVB Set Pulse Generator Width.vi"() -> ()  [unwired: 10 in, 2 out]
  n759 = call "RSZVB Get Pulse Generator Delay.vi"() -> ()  [unwired: 9 in, 3 out]
  n760 = call "RSZVB Set Harmonic Filter.vi"() -> ()  [unwired: 10 in, 2 out]
  n761 = call "RSZVB Set Pulse Generator Assignment.vi"() -> ()  [unwired: 10 in, 2 out]
  n762 = call "RSZVB Set Fixed Power To Signal.vi"() -> ()  [unwired: 10 in, 2 out]
  n763 = call "RSZVB Set SAW Parallel L.vi"() -> ()  [unwired: 10 in, 2 out]
  n764 = call "RSZVB Get SAW Simulation Type.vi"() -> ()  [unwired: 9 in, 3 out]
  n765 = call "RSZVB Trace Rename.vi"() -> ()  [unwired: 10 in, 2 out]
  n766 = call "RSZVB Set Simultaneous Measurement Frequency Offset State.vi"() -> ()  [unwired: 10 in, 2 out]
  n767 = call "RSZVB Set Simultaneous Measurement Minimum Frequency Offset Direct.vi"() -> ()  [unwired: 10 in, 2 out]
  n768 = call "RSZVB Set Pulse Generator Mode.vi"() -> ()  [unwired: 10 in, 2 out]
  n769 = call "RSZVB Get Pulse Train Segment Start.vi"() -> ()  [unwired: 9 in, 3 out]
  n770 = call "RSZVB Set Fundamental Power Signal.vi"() -> ()  [unwired: 10 in, 2 out]
  n771 = call "RSZVB Set Sweep Meas Delay.vi"() -> ()  [unwired: 10 in, 2 out]
  n772 = call "RSZVB Set Fundamental Frequency Signal.vi"() -> ()  [unwired: 10 in, 2 out]
  n773 = call "RSZVB Set Fixed Frequency.vi"() -> ()  [unwired: 10 in, 2 out]
  n774 = call "RSZVB Set Frequency Conversion Mode Stage 2.vi"() -> ()  [unwired: 10 in, 2 out]
  n775 = call "RSZVB Set Frequency RF Conversion Factor.vi"() -> ()  [unwired: 10 in, 2 out]
  n776 = call "RSZVB Get Coherent Signal Amplitude.vi"() -> ()  [unwired: 9 in, 3 out]
  n777 = call "RSZVB Select More Ratios Generator.vi"() -> ()  [unwired: 14 in, 2 out]
  n778 = call "RSZVB Trace Add S-Parameter Group.vi"() -> ()  [unwired: 10 in, 2 out]
  n779 = call "RSZVB Trace Select.vi"() -> ()  [unwired: 10 in, 2 out]
  n780 = call "RSZVB Get Generator Step Attenuators.vi"() -> ()  [unwired: 9 in, 3 out]
  n781 = call "RSZVB Set RF State.vi"() -> ()  [unwired: 10 in, 2 out]
  n782 = call "RSZVB Set Meas Bandwidth Reduction.vi"() -> ()  [unwired: 10 in, 2 out]
  n783 = call "RSZVB Get Current Sweep.vi"() -> ()  [unwired: 9 in, 3 out]
  n784 = call "RSZVB Set Converter Cal Power Offset.vi"() -> ()  [unwired: 10 in, 2 out]
  n785 = call "RSZVB Set Type Of Advanced Power Transfer Model.vi"() -> ()  [unwired: 10 in, 2 out]
  n786 = call "RSZVB Set Converter Port Assignment.vi"() -> ()  [unwired: 10 in, 2 out]
  n787 = call "RSZVB Get Port Waveguide Attenuator.vi"() -> ()  [unwired: 9 in, 3 out]
  n788 = call "RSZVB Get Port Electronic Power Treshold.vi"() -> ()  [unwired: 9 in, 3 out]
  n789 = call "RSZVB Get Power Meter Frequency Conversion.vi"() -> ()  [unwired: 6 in, 6 out]
  n790 = call "RSZVB Get Measure A Waves State.vi"() -> ()  [unwired: 9 in, 3 out]
  n791 = call "RSZVB Get Logical Port Common Ref Impedance.vi"() -> ()  [unwired: 8 in, 4 out]
  n792 = call "RSZVB Get Physical Port Ref Impedance.vi"() -> ()  [unwired: 8 in, 4 out]
  n793 = call "RSZVB Get RF Signal Source State.vi"() -> ()  [unwired: 9 in, 3 out]
  n794 = call "RSZVB Get Port Power Generator Offset.vi"() -> ()  [unwired: 8 in, 4 out]
  n795 = call "RSZVB Get TDIF Amplitude Imbalance Logical Port.vi"() -> ()  [unwired: 9 in, 3 out]
  n796 = call "RSZVB Set TDIF Phase Imbalance Logical Port.vi"() -> ()  [unwired: 10 in, 2 out]
  n797 = call "RSZVB Get TDIF Phase Imbalance Stop Phase.vi"() -> ()  [unwired: 9 in, 3 out]
  n798 = call "RSZVB Set TDIF Receiver Frequency.vi"() -> ()  [unwired: 10 in, 2 out]
  n799 = call "RSZVB Trace Export Data With Options Extended.vi"() -> ()  [unwired: 10 in, 2 out]
  n800 = call "RSZVB Trace Export Data Ports Incomplete.vi"() -> ()  [unwired: 14 in, 2 out]
  n801 = call "RSZVB Get Linearity Deviation State.vi"() -> ()  [unwired: 9 in, 3 out]
  n802 = call "RSZVB Set Linearity Deviation Constant.vi"() -> ()  [unwired: 10 in, 2 out]
  n803 = call "RSZVB Get Generator Port Resolution Bandwidth.vi"() -> ()  [unwired: 9 in, 3 out]
  n804 = call "RSZVB Set Trigger Delay.vi"() -> ()  [unwired: 10 in, 2 out]
  n805 = call "RSZVB Get Generator Port Trigger Delay.vi"() -> ()  [unwired: 9 in, 3 out]
  n806 = call "RSZVB Set Trigger On.vi"() -> ()  [unwired: 10 in, 2 out]
  n807 = call "RSZVB Get IMOD Upper Tone Source.vi"() -> ()  [unwired: 8 in, 4 out]
  n808 = call "RSZVB Get IMOD Measurement Order.vi"() -> ()  [unwired: 9 in, 3 out]
  n809 = call "RSZVB Get IMOD Distortion Measurement Calibration State.vi"() -> ()  [unwired: 9 in, 3 out]
  n810 = call "RSZVB Get Noise Figure Measurement Mode.vi"() -> ()  [unwired: 9 in, 3 out]
  n811 = call "RSZVB Get Noise Figure RF Image Correction.vi"() -> ()  [unwired: 9 in, 3 out]
  n812 = call "RSZVB Get Virtual Transform Balanced Port.vi"() -> ()  [unwired: 9 in, 3 out]
  n813 = call "RSZVB Get Virtual Transform Single Ended State.vi"() -> ()  [unwired: 9 in, 3 out]
  n814 = call "RSZVB Load And Interchange Single Ended Port Circuit Model Data.vi"() -> ()  [unwired: 10 in, 2 out]
  n815 = call "RSZVB Get Virtual Transform Ground Loop Circuit Model.vi"() -> ()  [unwired: 9 in, 3 out]
  n816 = call "RSZVB Set Virtual Transform Port Pair Circuit Model.vi"() -> ()  [unwired: 10 in, 2 out]
  n817 = call "RSZVB Get Time Gate Stop Time.vi"() -> ()  [unwired: 9 in, 3 out]
  n818 = call "RSZVB Set Time Gate Filter.vi"() -> ()  [unwired: 10 in, 2 out]
  n819 = call "RSZVB Get Time Gate Shape.vi"() -> ()  [unwired: 9 in, 3 out]
  n820 = call "RSZVB Trace Complex Response Data.vi"() -> ()  [unwired: 9 in, 3 out]
  n821 = call "RSZVB Trace Stimulus Data.vi"() -> ()  [unwired: 9 in, 3 out]
  n822 = call "RSZVB Trace Stimulus Data ZVR.vi"() -> ()  [unwired: 9 in, 3 out]
  n823 = call "RSZVB Get Frequency Step Size.vi"() -> ()  [unwired: 9 in, 3 out]
  n824 = call "RSZVB Configure Trigger RF Power.vi"() -> ()  [unwired: 10 in, 2 out]
  n825 = call "RSZVB Get IMOD Two Tone Output.vi"() -> ()  [unwired: 9 in, 3 out]
  n826 = call "RSZVB Terminate Noise Figure Calibration.vi"() -> ()  [unwired: 10 in, 2 out]
  n827 = call "RSZVB Get Marker Search Mode.vi"() -> ()  [unwired: 9 in, 3 out]
  n828 = call "RSZVB Get Limit Line Fail Beep.vi"() -> ()  [unwired: 9 in, 3 out]
  n829 = call "RSZVB Write Limit Line Segment List.vi"() -> ()  [unwired: 14 in, 2 out]
  n830 = call "RSZVB Save Limit Line.vi"() -> ()  [unwired: 10 in, 2 out]
  n831 = call "RSZVB Set Limit Domain Units.vi"() -> ()  [unwired: 10 in, 2 out]
  n832 = call "RSZVB Set Center Frequency.vi"() -> ()  [unwired: 10 in, 2 out]
  n833 = call "RSZVB Set CW Frequency.vi"() -> ()  [unwired: 10 in, 2 out]
  n834 = call "RSZVB Set Source Port.vi"() -> ()  [unwired: 10 in, 2 out]
  n835 = call "RSZVB Send Trigger and Wait for OPC.vi"() -> ()  [unwired: 10 in, 2 out]
  n836 = call "RSZVB Delete Balanced Port.vi"() -> ()  [unwired: 10 in, 2 out]
  n837 = call "RSZVB Get Differential Mode Impedance.vi"() -> ()  [unwired: 9 in, 3 out]
  n838 = call "RSZVB Set Time Domain Stop Time.vi"() -> ()  [unwired: 10 in, 2 out]
  n839 = call "RSZVB Set Time Domain Time Span.vi"() -> ()  [unwired: 10 in, 2 out]
  n840 = call "RSZVB Set Time Domain Transformation Filter.vi"() -> ()  [unwired: 10 in, 2 out]
  n841 = call "RSZVB Set Time Domain Transformation Resolution Efactor.vi"() -> ()  [unwired: 10 in, 2 out]
  n842 = call "RSZVB Set DC Value.vi"() -> ()  [unwired: 10 in, 2 out]
  n843 = call "RSZVB Get Continuous Extrapolation.vi"() -> ()  [unwired: 9 in, 3 out]
  n844 = call "RSZVB Get Marker Response.vi"() -> ()  [unwired: 9 in, 3 out]
  n845 = call "RSZVB Get Reference Marker Response.vi"() -> ()  [unwired: 9 in, 3 out]
  n846 = call "RSZVB Set Delta Marker State.vi"() -> ()  [unwired: 10 in, 2 out]
  n847 = call "RSZVB Get Discrete Marker.vi"() -> ()  [unwired: 9 in, 3 out]
  n848 = call "RSZVB Set All Markers Off.vi"() -> ()  [unwired: 10 in, 2 out]
  n849 = call "RSZVB Set Port Configuration.vi"() -> ()  [unwired: 10 in, 2 out]
  n850 = call "RSZVB Set Aperture Group Delay Steps.vi"() -> ()  [unwired: 10 in, 2 out]
  n851 = call "RSZVB Set Trace Scale Divisions.vi"() -> ()  [unwired: 10 in, 2 out]
  n852 = call "RSZVB Set Trace Ref Position.vi"() -> ()  [unwired: 10 in, 2 out]
  n853 = call "RSZVB Set Trace Math Function.vi"() -> ()  [unwired: 10 in, 2 out]
  n854 = call "RSZVB Get Trace Transform Conversion.vi"() -> ()  [unwired: 9 in, 3 out]
  n855 = call "RSZVB Marker Bandfilter Results ZVR.vi"() -> ()  [unwired: 9 in, 3 out]
  n856 = call "RSZVB Set Power Stimulus.vi"() -> ()  [unwired: 10 in, 2 out]
  n857 = call "RSZVB Get TRM Combiner State.vi"() -> ()  [unwired: 9 in, 3 out]
  n858 = call "RSZVB Set TRM User Source Path Extension State.vi"() -> ()  [unwired: 10 in, 2 out]
  n859 = call "RSZVB Get TRM Pulse Modulator Source.vi"() -> ()  [unwired: 9 in, 3 out]
  n860 = call "RSZVB Get TRM Number Of Units.vi"() -> ()  [unwired: 9 in, 3 out]
  n861 = call "RSZVB Define Group Of All Measured Ports.vi"() -> ()  [unwired: 10 in, 2 out]
  n862 = call "RSZVB Get UI Signal Pin 20.vi"() -> ()  [unwired: 9 in, 3 out]
  n863 = call "RSZVB Get UI Port Next State.vi"() -> ()  [unwired: 9 in, 3 out]
  n864 = call "RSZVB Define Pulse Train Segments.vi"() -> ()  [unwired: 10 in, 2 out]
  n865 = call "RSZVB Get Frequency Info.vi"() -> ()  [unwired: 9 in, 3 out]
  n866 = call "RSZVB Get Marker Color State.vi"() -> ()  [unwired: 9 in, 3 out]
  n867 = call "RSZVB Trace Get RGB Color.vi"() -> ()  [unwired: 9 in, 7 out]
  n868 = call "RSZVB Calibration Standards Catalog.vi"() -> ()  [unwired: 9 in, 3 out]
  n869 = call "RSZVB Diagram Area Catalog.vi"() -> ()  [unwired: 9 in, 3 out]
  n870 = call "RSZVB Get Analyzer Hostname.vi"() -> ()  [unwired: 9 in, 3 out]
  n871 = call "RSZVB Get Power Port Limit Direct Generator And Receiver State.vi"() -> ()  [unwired: 9 in, 3 out]
  n872 = call "RSZVB Set Remote Language.vi"() -> ()  [unwired: 10 in, 2 out]
  n873 = call "RSZVB Delete External Generator.vi"() -> ()  [unwired: 10 in, 2 out]
  n874 = call "RSZVB Set Auto Config NRPZxx.vi"() -> ()  [unwired: 10 in, 2 out]
  n875 = call "RSZVB Get Restart Behavior.vi"() -> ()  [unwired: 9 in, 3 out]
  n876 = call "RSZVB Get Error Display State.vi"() -> ()  [unwired: 9 in, 3 out]
  n877 = call "RSZVB Get Fast Multiport Correction.vi"() -> ()  [unwired: 9 in, 3 out]
  n878 = call "RSZVB Query Extension Unit Hardware Options.vi"() -> ()  [unwired: 9 in, 3 out]
  n879 = call "RSZVB Get Calculation of Bandfilter Center Frequency.vi"() -> ()  [unwired: 9 in, 3 out]
  n880 = call "RSZVB Get Calibration Kit User Connector Type.vi"() -> ()  [unwired: 9 in, 3 out]
  n881 = call "RSZVB Delete Calibration Kit.vi"() -> ()  [unwired: 10 in, 2 out]
  n882 = call "RSZVB Set Loss Reference Frequency.vi"() -> ()  [unwired: 10 in, 2 out]
  n883 = call "RSZVB Get Fixture Compensation Auto Length And Loss Calculation.vi"() -> ()  [unwired: 9 in, 3 out]
  n884 = call "RSZVB Getting Started.vi"() -> ()  [unwired: 12 in]
  n885 = call "RSZVB Set Same Connector Gender at All Ports.vi"() -> ()  [unwired: 10 in, 2 out]
  n886 = call "RSZVB Set S-Parameter Detector.vi"() -> ()  [unwired: 10 in, 2 out]
  n887 = call "RSZVB Set Ripple Limit Response Domain Format Units.vi"() -> ()  [unwired: 10 in, 2 out]
  n888 = call "RSZVB Get Source Power Calibration Paramater Stop.vi"() -> ()  [unwired: 9 in, 3 out]
  n889 = call "RSZVB Write Receiver Power Correction Data.vi"() -> ()  [unwired: 10 in, 2 out]
  n890 = call "RSZVB Get Calibration Connection.vi"() -> ()  [unwired: 6 in, 6 out]
  n891 = call "RSZVB Get Calibration Data Timestamp.vi"() -> ()  [unwired: 9 in, 3 out]
  n892 = call "RSZVB Configure Calibration Unit Standard.vi"() -> ()  [unwired: 10 in, 2 out]
  n893 = call "RSZVB Get Load Matching Correction.vi"() -> ()  [unwired: 9 in, 3 out]
  n894 = call "RSZVB Get Source Power Calibration Convergence Factor.vi"() -> ()  [unwired: 9 in, 3 out]
  n895 = call "RSZVB Set Two Port Transmission Coefficients Enabled.vi"() -> ()  [unwired: 10 in, 2 out]
  n896 = call "RSZVB Get Power Loss List Coefficient.vi"() -> ()  [unwired: 8 in, 4 out]
  n897 = call "RSZVB Calibration Auto Assignment Save.vi"() -> ()  [unwired: 10 in, 2 out]
  n898 = call "RSZVB Export Characterization Data to Touchstone Files.vi"() -> ()  [unwired: 10 in, 2 out]
  n899 = call "RSZVB Get Calibration Date.vi"() -> ()  [unwired: 9 in, 3 out]
  n900 = call "RSZVB Get Calibration Data Bandwidth.vi"() -> ()  [unwired: 9 in, 3 out]
  n901 = call "RSZVB Marker Search Results.vi"() -> ()  [unwired: 8 in, 4 out]
  n902 = call "RSZVB Set A Wave Ideal Power Meter Match State.vi"() -> ()  [unwired: 10 in, 2 out]
  n903 = call "RSZVB Calibration Manager.vi"() -> ()  [unwired: 10 in, 2 out]
  n904 = call "RSZVB Set PI Controller Integration Time.vi"() -> ()  [unwired: 10 in, 2 out]
  n905 = call "RSZVB Get Source Power Calibration Generator State.vi"() -> ()  [unwired: 9 in, 3 out]
  n906 = call "RSZVB Generator Power Calibration Harmonic.vi"() -> ()  [unwired: 10 in, 2 out]
  n907 = call "RSZVB Get Reference Receiver Calibration State.vi"() -> ()  [unwired: 9 in, 3 out]
  n908 = call "RSZVB Get Dummy Source Power Calibration State.vi"() -> ()  [unwired: 9 in, 3 out]
  n909 = call "RSZVB Get Number Of Readings.vi"() -> ()  [unwired: 9 in, 3 out]
  n910 = call "RSZVB Get Other Sources State.vi"() -> ()  [unwired: 9 in, 3 out]
  n911 = call "RSZVB Get Calibration Power Offset.vi"() -> ()  [unwired: 9 in, 3 out]
  n912 = call "RSZVB Get Reference Receiver After First Cal Sweep.vi"() -> ()  [unwired: 9 in, 3 out]
  n913 = call "RSZVB Get Calibration Power Meter Readings.vi"() -> ()  [unwired: 9 in, 3 out]
  n914 = call "RSZVB Set Correction State.vi"() -> ()  [unwired: 10 in, 2 out]
  n915 = call "RSZVB Set Trace Compression Value.vi"() -> ()  [unwired: 10 in, 2 out]
  n916 = call "RSZVB Get Renormalization Mode.vi"() -> ()  [unwired: 9 in, 3 out]
  n917 = call "RSZVB Start Calibration With Options.vi"() -> ()  [unwired: 14 in, 2 out]
  n918 = call "RSZVB Save Calibration Data.vi"() -> ()  [unwired: 10 in, 2 out]
  n919 = call "RSZVB Get Internal Signal Source.vi"() -> ()  [unwired: 9 in, 3 out]
  n920 = call "RSZVB Get Harmonic Order.vi"() -> ()  [unwired: 9 in, 3 out]
  n921 = call "RSZVB Set Harmonic Relative State.vi"() -> ()  [unwired: 10 in, 2 out]
  n922 = call "RSZVB Get Signal Source.vi"() -> ()  [unwired: 8 in, 4 out]
  n923 = call "RSZVB IF Receiver Calibration.vi"() -> ()  [unwired: 10 in, 2 out]
  n924 = call "RSZVB Get Mixer Delay LAN Connection.vi"() -> ()  [unwired: 9 in, 3 out]
  n925 = call "RSZVB Get Mixer Delay Aperture.vi"() -> ()  [unwired: 9 in, 3 out]
  n926 = call "RSZVB Set Mixer Delay Division By Two Enabled.vi"() -> ()  [unwired: 10 in, 2 out]
  n927 = call "RSZVB Get Mixer Delay Correction.vi"() -> ()  [unwired: 9 in, 3 out]
  n928 = call "RSZVB Get Internal Signal Source AUX.vi"() -> ()  [unwired: 9 in, 3 out]
  n929 = call "RSZVB Set AUX Fixed Power.vi"() -> ()  [unwired: 10 in, 2 out]
  n930 = call "RSZVB Set Automatic Level Control State.vi"() -> ()  [unwired: 10 in, 2 out]
  n931 = call "RSZVB Set ALC Port Clamp.vi"() -> ()  [unwired: 10 in, 2 out]
  n932 = call "RSZVB Set ALC Port Coupling.vi"() -> ()  [unwired: 10 in, 2 out]
  n933 = call "RSZVB Set ALC Port Offset State.vi"() -> ()  [unwired: 10 in, 2 out]
  n934 = call "RSZVB Set ALC Port Setting Tolerance.vi"() -> ()  [unwired: 10 in, 2 out]
  n935 = call "RSZVB Set Chopped Pulse Profile Mode.vi"() -> ()  [unwired: 10 in, 2 out]
  n936 = call "RSZVB Get Harmonic Filter.vi"() -> ()  [unwired: 9 in, 3 out]
  n937 = call "RSZVB Get Pulse Generator Assignment.vi"() -> ()  [unwired: 9 in, 3 out]
  n938 = call "RSZVB Store Mixer Delay Calibration Data.vi"() -> ()  [unwired: 10 in, 2 out]
  n939 = call "RSZVB Get SAW Parallel L.vi"() -> ()  [unwired: 9 in, 3 out]
  n940 = call "RSZVB Get Simultaneous Measurement Frequency Offset State.vi"() -> ()  [unwired: 9 in, 3 out]
  n941 = call "RSZVB Get Simultaneous Measurement Minimum Frequency Offset Direct.vi"() -> ()  [unwired: 9 in, 3 out]
  n942 = call "RSZVB Get Pulse Generator Width.vi"() -> ()  [unwired: 9 in, 3 out]
  n943 = call "RSZVB Get Pulse Generator Mode.vi"() -> ()  [unwired: 9 in, 3 out]
  n944 = call "RSZVB Set Pulse Train Segment Stop.vi"() -> ()  [unwired: 10 in, 2 out]
  n945 = call "RSZVB Trace List Catalog.vi"() -> ()  [unwired: 9 in, 3 out]
  n946 = call "RSZVB Set Physical Port Resolution Bandwidth.vi"() -> ()  [unwired: 10 in, 2 out]
  n947 = call "RSZVB Load Segment.vi"() -> ()  [unwired: 10 in, 2 out]
  n948 = call "RSZVB Set Generator Frequency Conversion.vi"() -> ()  [unwired: 18 in, 2 out]
  n949 = call "RSZVB Set Local Oscilator A State.vi"() -> ()  [unwired: 10 in, 2 out]
  n950 = call "RSZVB Set Logical Port Differential Ref Impedance.vi"() -> ()  [unwired: 10 in, 2 out]
  n951 = call "RSZVB Set IF Gain.vi"() -> ()  [unwired: 10 in, 2 out]
  n952 = call "RSZVB Set Permanent Signal Source State.vi"() -> ()  [unwired: 10 in, 2 out]
  n953 = call "RSZVB Set Slope.vi"() -> ()  [unwired: 10 in, 2 out]
  n954 = call "RSZVB Set TDIF Amplitude Imbalance Start Power.vi"() -> ()  [unwired: 10 in, 2 out]
  n955 = call "RSZVB Get TDIF Phase Imbalance Logical Port.vi"() -> ()  [unwired: 9 in, 3 out]
  n956 = call "RSZVB Set TDIF Source Power Mode.vi"() -> ()  [unwired: 10 in, 2 out]
  n957 = call "RSZVB Get TDIF Receiver Frequency.vi"() -> ()  [unwired: 9 in, 3 out]
  n958 = call "RSZVB Get Fundamental Power Signal.vi"() -> ()  [unwired: 9 in, 3 out]
  n959 = call "RSZVB Get Fixed Power To Signal.vi"() -> ()  [unwired: 9 in, 3 out]
  n960 = call "RSZVB Select More Ratios Generator With Detector.vi"() -> ()  [unwired: 14 in, 2 out]
  n961 = call "RSZVB Channel Trace Export Data.vi"() -> ()  [unwired: 10 in, 2 out]
  n962 = call "RSZVB Delete Selected Segment.vi"() -> ()  [unwired: 10 in, 2 out]
  n963 = call "RSZVB Get Sweep Segment Start Frequency.vi"() -> ()  [unwired: 9 in, 3 out]
  n964 = call "RSZVB Get Sweep Segment Name.vi"() -> ()  [unwired: 9 in, 3 out]
  n965 = call "RSZVB Get Sweep Segment Meas Bandwidth.vi"() -> ()  [unwired: 9 in, 3 out]
  n966 = call "RSZVB Get Sweep Segment Independent Spur Avoid.vi"() -> ()  [unwired: 9 in, 3 out]
  n967 = call "RSZVB Get Sweep Segment Sweep Time.vi"() -> ()  [unwired: 9 in, 3 out]
  n968 = call "RSZVB Get Sweep Segment Independent Point Delay.vi"() -> ()  [unwired: 9 in, 3 out]
  n969 = call "RSZVB Get Sweep Segment Bits State.vi"() -> ()  [unwired: 9 in, 3 out]
  n970 = call "RSZVB Get Converter Cal Power Offset.vi"() -> ()  [unwired: 9 in, 3 out]
  n971 = call "RSZVB Get Type Of Advanced Power Transfer Model.vi"() -> ()  [unwired: 9 in, 3 out]
  n972 = call "RSZVB Get Converter Port Assignment.vi"() -> ()  [unwired: 9 in, 3 out]
  n973 = call "RSZVB Set Port Waveguide Attenuator Slope.vi"() -> ()  [unwired: 10 in, 2 out]
  n974 = call "RSZVB Set Port Electronic Power Reduction.vi"() -> ()  [unwired: 10 in, 2 out]
  n975 = call "RSZVB Get Fundamental Frequency Signal.vi"() -> ()  [unwired: 9 in, 3 out]
  n976 = call "RSZVB Get Frequency Conversion Mode Stage 2.vi"() -> ()  [unwired: 9 in, 3 out]
  n977 = call "RSZVB Get Frequency RF Conversion Factor.vi"() -> ()  [unwired: 8 in, 4 out]
  n978 = call "RSZVB Get Pulse Time Stop.vi"() -> ()  [unwired: 9 in, 3 out]
  n979 = call "RSZVB Get Pulse Evaluation Mode.vi"() -> ()  [unwired: 9 in, 3 out]
  n980 = call "RSZVB Get Pulse Section Limit Lines State.vi"() -> ()  [unwired: 9 in, 3 out]
  n981 = call "RSZVB Get Fixed Frequency.vi"() -> ()  [unwired: 9 in, 3 out]
  n982 = call "RSZVB Set Coherent Signal Phase.vi"() -> ()  [unwired: 10 in, 2 out]
  n983 = call "RSZVB Trace Complex Response Catalog.vi"() -> ()  [unwired: 9 in, 3 out]
  n984 = call "RSZVB Write Memory Trace Data.vi"() -> ()  [unwired: 10 in, 2 out]
  n985 = call "RSZVB Trace Response Data S-Parameter Group.vi"() -> ()  [unwired: 9 in, 3 out]
  n986 = call "RSZVB Query Trace Add S-Parameter Group.vi"() -> ()  [unwired: 9 in, 3 out]
  n987 = call "RSZVB Trace Delete.vi"() -> ()  [unwired: 10 in, 2 out]
  n988 = call "RSZVB Get Linearity Deviation Constant.vi"() -> ()  [unwired: 9 in, 3 out]
  n989 = call "RSZVB Marker Bandfilter Tracking.vi"() -> ()  [unwired: 10 in, 2 out]
  n990 = call "RSZVB Set Automatic Generator Attenuator.vi"() -> ()  [unwired: 10 in, 2 out]
  n991 = call "RSZVB Get RF State.vi"() -> ()  [unwired: 9 in, 3 out]
  n992 = call "RSZVB Get Meas Bandwidth Reduction.vi"() -> ()  [unwired: 9 in, 3 out]
  n993 = call "RSZVB Restart Average.vi"() -> ()  [unwired: 10 in, 2 out]
  n994 = call "RSZVB Get Trigger Delay.vi"() -> ()  [unwired: 9 in, 3 out]
  n995 = call "RSZVB Set Physical Port Trigger Delay.vi"() -> ()  [unwired: 10 in, 2 out]
  n996 = call "RSZVB Get Trigger On.vi"() -> ()  [unwired: 9 in, 3 out]
  n997 = call "RSZVB Set IMOD Tone Distance.vi"() -> ()  [unwired: 10 in, 2 out]
  n998 = call "RSZVB Set IMOD Internal Combiner.vi"() -> ()  [unwired: 10 in, 2 out]
  n999 = call "RSZVB Start IMOD Lower Tone Source Power Calibration.vi"() -> ()  [unwired: 10 in, 2 out]
  n1000 = call "RSZVB Disable IMOD Measurement.vi"() -> ()  [unwired: 10 in, 2 out]
  n1001 = call "RSZVB Set Noise Figure LO Oscillator.vi"() -> ()  [unwired: 10 in, 2 out]
  n1002 = call "RSZVB Set Sweep Count.vi"() -> ()  [unwired: 10 in, 2 out]
  n1003 = call "RSZVB Get Sweep Meas Delay.vi"() -> ()  [unwired: 9 in, 3 out]
  n1004 = call "RSZVB Set Noise Figure Calibration State.vi"() -> ()  [unwired: 10 in, 2 out]
  n1005 = call "RSZVB Complete Noise Figure Calibration.vi"() -> ()  [unwired: 10 in, 2 out]
  n1006 = call "RSZVB Set Virtual Transform Balanced Circuit Model.vi"() -> ()  [unwired: 10 in, 2 out]
  n1007 = call "RSZVB Set Virtual Transform Single Ended Port.vi"() -> ()  [unwired: 14 in, 2 out]
  n1008 = call "RSZVB Set Virtual Transform Ground Loop State.vi"() -> ()  [unwired: 10 in, 2 out]
  n1009 = call "RSZVB Load Ground Loop Circuit Model Data.vi"() -> ()  [unwired: 10 in, 2 out]
  n1010 = call "RSZVB Get Virtual Transform Port Pair Circuit Model.vi"() -> ()  [unwired: 9 in, 3 out]
  n1011 = call "RSZVB Get Aperture Group Delay Steps.vi"() -> ()  [unwired: 9 in, 3 out]
  n1012 = call "RSZVB Set Trace Scale Divisions By Name.vi"() -> ()  [unwired: 10 in, 2 out]
  n1013 = call "RSZVB Set Trace Ref Position By Name.vi"() -> ()  [unwired: 10 in, 2 out]
  n1014 = call "RSZVB Get Time Domain Stop Time.vi"() -> ()  [unwired: 9 in, 3 out]
  n1015 = call "RSZVB Get Time Domain Time Span.vi"() -> ()  [unwired: 9 in, 3 out]
  n1016 = call "RSZVB Get Time Domain Transformation Filter.vi"() -> ()  [unwired: 9 in, 3 out]
  n1017 = call "RSZVB Get Time Domain Transformation Resolution Efactor.vi"() -> ()  [unwired: 9 in, 3 out]
  n1018 = call "RSZVB Get DC Value.vi"() -> ()  [unwired: 9 in, 3 out]
  n1019 = call "RSZVB Calculate Harmonic Grid.vi"() -> ()  [unwired: 10 in, 2 out]
  n1020 = call "RSZVB Set Time Gate Center Time.vi"() -> ()  [unwired: 10 in, 2 out]
  n1021 = call "RSZVB Get Time Gate Filter.vi"() -> ()  [unwired: 9 in, 3 out]
  n1022 = call "RSZVB Set Time Gate Span.vi"() -> ()  [unwired: 10 in, 2 out]
  n1023 = call "RSZVB Set Marker Search Result State.vi"() -> ()  [unwired: 10 in, 2 out]
  n1024 = call "RSZVB Get Limit Check Result.vi"() -> ()  [unwired: 9 in, 3 out]
  n1025 = call "RSZVB Shift Limit Line Segment List.vi"() -> ()  [unwired: 10 in, 2 out]
  n1026 = call "RSZVB Import Trace as Limit Line.vi"() -> ()  [unwired: 10 in, 2 out]
  n1027 = call "RSZVB Set Limit Response Domain Complex Units.vi"() -> ()  [unwired: 10 in, 2 out]
  n1028 = call "RSZVB Set Sweep Single - All Chans.vi"() -> ()  [unwired: 10 in, 2 out]
  n1029 = call "RSZVB Configure Trigger Manual.vi"() -> ()  [unwired: 10 in, 2 out]
  n1030 = call "RSZVB Get Center Frequency.vi"() -> ()  [unwired: 9 in, 3 out]
  n1031 = call "RSZVB Get CW Frequency.vi"() -> ()  [unwired: 9 in, 3 out]
  n1032 = call "RSZVB Get Source Port.vi"() -> ()  [unwired: 9 in, 3 out]
  n1033 = call "RSZVB Get Port Configuration.vi"() -> ()  [unwired: 6 in, 6 out]
  n1034 = call "RSZVB Delete All Balanced Ports.vi"() -> ()  [unwired: 10 in, 2 out]
  n1035 = call "RSZVB Set Common Mode Impedance.vi"() -> ()  [unwired: 10 in, 2 out]
  n1036 = call "RSZVB Get Trace Math Function.vi"() -> ()  [unwired: 9 in, 3 out]
  n1037 = call "RSZVB Get Power Stimulus.vi"() -> ()  [unwired: 9 in, 3 out]
  n1038 = call "RSZVB Set TRM Power Amplifier State.vi"() -> ()  [unwired: 10 in, 2 out]
  n1039 = call "RSZVB Get TRM User Source Path Extension State.vi"() -> ()  [unwired: 9 in, 3 out]
  n1040 = call "RSZVB Set TRM Pulse Generator Source.vi"() -> ()  [unwired: 10 in, 2 out]
  n1041 = call "RSZVB Get TRM Unit Device ID.vi"() -> ()  [unwired: 9 in, 3 out]
  n1042 = call "RSZVB Get Group Of All Measured Ports.vi"() -> ()  [unwired: 9 in, 3 out]
  n1043 = call "RSZVB Configure Chopped Pulse Profile.vi"() -> ()  [unwired: 10 in, 2 out]
  n1044 = call "RSZVB Trace Diagram Area Catalog.vi"() -> ()  [unwired: 9 in, 3 out]
  n1045 = call "RSZVB Get Same Connector Gender at All Ports.vi"() -> ()  [unwired: 9 in, 3 out]
  n1046 = call "RSZVB Get S-Parameter Detector.vi"() -> ()  [unwired: 9 in, 3 out]
  n1047 = call "RSZVB Calibration Standards Catalog With Label.vi"() -> ()  [unwired: 9 in, 3 out]
  n1048 = call "RSZVB Delete Calibration Kit With Label.vi"() -> ()  [unwired: 10 in, 2 out]
  n1049 = call "RSZVB Get Loss Reference Frequency.vi"() -> ()  [unwired: 9 in, 3 out]
  n1050 = call "RSZVB Get PI Controller Integration Time.vi"() -> ()  [unwired: 9 in, 3 out]
  n1051 = call "RSZVB Set Calibration Kit User Connector Type With Label.vi"() -> ()  [unwired: 10 in, 2 out]
  n1052 = call "RSZVB Get Source Power Calibration Paramater Points.vi"() -> ()  [unwired: 9 in, 3 out]
  n1053 = call "RSZVB Get A Wave Ideal Power Meter Match State.vi"() -> ()  [unwired: 9 in, 3 out]
  n1054 = call "RSZVB Receiver Power Calibration Harmonic.vi"() -> ()  [unwired: 10 in, 2 out]
  n1055 = call "RSZVB Calibration Auto with Timeout.vi"() -> ()  [unwired: 18 in, 2 out]
  n1056 = call "RSZVB Calibration Auto Assignments Delete All.vi"() -> ()  [unwired: 10 in, 2 out]
  n1057 = call "RSZVB Set Active Calibration Unit.vi"() -> ()  [unwired: 10 in, 2 out]
  n1058 = call "RSZVB Set Factory Calibration State.vi"() -> ()  [unwired: 10 in, 2 out]
  n1059 = call "RSZVB Set Calibration Correction Base Frequency State.vi"() -> ()  [unwired: 10 in, 2 out]
  n1060 = call "RSZVB Set Source Power Calibration Sensitivity Correction Range.vi"() -> ()  [unwired: 10 in, 2 out]
  n1061 = call "RSZVB Calibration Auto.vi"() -> ()  [unwired: 18 in, 2 out]
  n1062 = call "RSZVB Export User Characterization Data to Touchstone Files.vi"() -> ()  [unwired: 10 in, 2 out]
  n1063 = call "RSZVB Get Calibration State.vi"() -> ()  [unwired: 9 in, 3 out]
  n1064 = call "RSZVB Get Calibration Data Point Delay.vi"() -> ()  [unwired: 9 in, 3 out]
  n1065 = call "RSZVB Set LN Preamplifier.vi"() -> ()  [unwired: 10 in, 2 out]
  n1066 = call "RSZVB Set Tolerance.vi"() -> ()  [unwired: 10 in, 2 out]
  n1067 = call "RSZVB Set Port Power Offset.vi"() -> ()  [unwired: 10 in, 2 out]
  n1068 = call "RSZVB Set Calibration Power Generator Offset.vi"() -> ()  [unwired: 10 in, 2 out]
  n1069 = call "RSZVB Set Power Calibration Method Source.vi"() -> ()  [unwired: 10 in, 2 out]
  n1070 = call "RSZVB Set SAW Serial C.vi"() -> ()  [unwired: 10 in, 2 out]
  n1071 = call "RSZVB Get Physical Port Resolution Bandwidth.vi"() -> ()  [unwired: 9 in, 3 out]
  n1072 = call "RSZVB Set Pulse Generator Single Period.vi"() -> ()  [unwired: 10 in, 2 out]
  n1073 = call "RSZVB Set Pulse Generator Master Channel.vi"() -> ()  [unwired: 10 in, 2 out]
  n1074 = call "RSZVB Set External Signal Generator Output.vi"() -> ()  [unwired: 10 in, 2 out]
  n1075 = call "RSZVB Set External Signal Source.vi"() -> ()  [unwired: 10 in, 2 out]
  n1076 = call "RSZVB LO Source Calibration.vi"() -> ()  [unwired: 10 in, 2 out]
  n1077 = call "RSZVB Define Mixer Delay Receiver.vi"() -> ()  [unwired: 10 in, 2 out]
  n1078 = call "RSZVB Set Mixer Delay Constant.vi"() -> ()  [unwired: 10 in, 2 out]
  n1079 = call "RSZVB Get Mixer Delay Division By Two Enabled.vi"() -> ()  [unwired: 9 in, 3 out]
  n1080 = call "RSZVB Set Mixer Delay Upper Tone Source.vi"() -> ()  [unwired: 10 in, 2 out]
  n1081 = call "RSZVB Set External Signal Source AUX.vi"() -> ()  [unwired: 10 in, 2 out]
  n1082 = call "RSZVB Get AUX Fixed Power.vi"() -> ()  [unwired: 9 in, 3 out]
  n1083 = call "RSZVB Set Simultaneous Measurement Minimum Frequency Offset Mode.vi"() -> ()  [unwired: 10 in, 2 out]
  n1084 = call "RSZVB Get Simultaneous Measurement Minimum Frequency Offset Operating Mode.vi"() -> ()  [unwired: 9 in, 3 out]
  n1085 = call "RSZVB Get Pulse Train Segment Stop.vi"() -> ()  [unwired: 9 in, 3 out]
  n1086 = call "RSZVB Get Chopped Pulse Profile Mode.vi"() -> ()  [unwired: 9 in, 3 out]
  n1087 = call "RSZVB Get Automatic Level Control State.vi"() -> ()  [unwired: 9 in, 3 out]
  n1088 = call "RSZVB Get ALC Port Clamp.vi"() -> ()  [unwired: 9 in, 3 out]
  n1089 = call "RSZVB Get ALC Port Coupling.vi"() -> ()  [unwired: 9 in, 3 out]
  n1090 = call "RSZVB Get ALC Port Offset State.vi"() -> ()  [unwired: 9 in, 3 out]
  n1091 = call "RSZVB Get ALC Port Setting Tolerance.vi"() -> ()  [unwired: 9 in, 3 out]
  n1092 = call "RSZVB Generate Default Calibration Data.vi"() -> ()  [unwired: 10 in, 2 out]
  n1093 = call "RSZVB Get Correction State.vi"() -> ()  [unwired: 9 in, 3 out]
  n1094 = call "RSZVB Set IF Signal Port.vi"() -> ()  [unwired: 10 in, 2 out]
  n1095 = call "RSZVB Set Calibration Reference Plane Shift.vi"() -> ()  [unwired: 10 in, 2 out]
  n1096 = call "RSZVB Set Advanced Power Transfer Model Frequency State.vi"() -> ()  [unwired: 10 in, 2 out]
  n1097 = call "RSZVB Set Converter Data Set Type.vi"() -> ()  [unwired: 10 in, 2 out]
  n1098 = call "RSZVB Set Port Transfer Model State.vi"() -> ()  [unwired: 10 in, 2 out]
  n1099 = call "RSZVB Get Port Waveguide Attenuator Slope.vi"() -> ()  [unwired: 9 in, 3 out]
  n1100 = call "RSZVB Get Port Electronic Power Reduction.vi"() -> ()  [unwired: 9 in, 3 out]
  n1101 = call "RSZVB Get Generator Frequency Conversion.vi"() -> ()  [unwired: 9 in, 7 out]
  n1102 = call "RSZVB Get Local Oscilator A State.vi"() -> ()  [unwired: 9 in, 3 out]
  n1103 = call "RSZVB Get Logical Port Differential Ref Impedance.vi"() -> ()  [unwired: 8 in, 4 out]
  n1104 = call "RSZVB Get IF Gain.vi"() -> ()  [unwired: 9 in, 3 out]
  n1105 = call "RSZVB Get Permanent Signal Source State.vi"() -> ()  [unwired: 9 in, 3 out]
  n1106 = call "RSZVB Get Slope.vi"() -> ()  [unwired: 9 in, 3 out]
  n1107 = call "RSZVB Set Harmonic Source Port.vi"() -> ()  [unwired: 10 in, 2 out]
  n1108 = call "RSZVB Get Harmonic Relative State.vi"() -> ()  [unwired: 9 in, 3 out]
  n1109 = call "RSZVB Set Signal Power Mode.vi"() -> ()  [unwired: 10 in, 2 out]
  n1110 = call "RSZVB Set Fixed Frequency Signal.vi"() -> ()  [unwired: 10 in, 2 out]
  n1111 = call "RSZVB Set Fixed Frequency To Signal.vi"() -> ()  [unwired: 10 in, 2 out]
  n1112 = call "RSZVB Extrapolate DC Value.vi"() -> ()  [unwired: 10 in, 2 out]
  n1113 = call "RSZVB Trace Response Single Sweep Data.vi"() -> ()  [unwired: 9 in, 3 out]
  n1114 = call "RSZVB Write Memory Trace Data Extended.vi"() -> ()  [unwired: 10 in, 2 out]
  n1115 = call "RSZVB Set Linearity Deviation Electrical Length.vi"() -> ()  [unwired: 10 in, 2 out]
  n1116 = call "RSZVB Set Sweep Segment Bit Values.vi"() -> ()  [unwired: 10 in, 2 out]
  n1117 = call "RSZVB Query Overlapping Sweep Segments.vi"() -> ()  [unwired: 9 in, 3 out]
  n1118 = call "RSZVB Set Fixed Power.vi"() -> ()  [unwired: 10 in, 2 out]
  n1119 = call "RSZVB Set Frequency High Accuracy.vi"() -> ()  [unwired: 10 in, 2 out]
  n1120 = call "RSZVB Set RF Image Frequency.vi"() -> ()  [unwired: 10 in, 2 out]
  n1121 = call "RSZVB Get Coherent Signal Phase.vi"() -> ()  [unwired: 9 in, 3 out]
  n1122 = call "RSZVB Delete All Segments.vi"() -> ()  [unwired: 10 in, 2 out]
  n1123 = call "RSZVB Set Sweep Segment Stop Frequency.vi"() -> ()  [unwired: 10 in, 2 out]
  n1124 = call "RSZVB Set Sweep Segment Power.vi"() -> ()  [unwired: 10 in, 2 out]
  n1125 = call "RSZVB Set Sweep Segment Independent Bandwidth.vi"() -> ()  [unwired: 10 in, 2 out]
  n1126 = call "RSZVB Set Sweep Segment Selectivity.vi"() -> ()  [unwired: 10 in, 2 out]
  n1127 = call "RSZVB Set Sweep Segment Independent Time.vi"() -> ()  [unwired: 10 in, 2 out]
  n1128 = call "RSZVB Set Sweep Segment Triggering.vi"() -> ()  [unwired: 10 in, 2 out]
  n1129 = call "RSZVB Set Pulse Time Bandwidth.vi"() -> ()  [unwired: 10 in, 2 out]
  n1130 = call "RSZVB Set Pulse Evaluation Section Start.vi"() -> ()  [unwired: 10 in, 2 out]
  n1131 = call "RSZVB Set Pulse Shift Stimulus.vi"() -> ()  [unwired: 10 in, 2 out]
  n1132 = call "RSZVB Set Partial Measurement Trigger Mode.vi"() -> ()  [unwired: 10 in, 2 out]
  n1133 = call "RSZVB Get Physical Port Trigger Delay.vi"() -> ()  [unwired: 9 in, 3 out]
  n1134 = call "RSZVB Set Trigger Period.vi"() -> ()  [unwired: 10 in, 2 out]
  n1135 = call "RSZVB Get Automatic Generator Attenuator.vi"() -> ()  [unwired: 9 in, 3 out]
  n1136 = call "RSZVB Set Meas Bandwidth.vi"() -> ()  [unwired: 10 in, 2 out]
  n1137 = call "RSZVB Set Average State.vi"() -> ()  [unwired: 10 in, 2 out]
  n1138 = call "RSZVB Get IMOD Tone Distance.vi"() -> ()  [unwired: 9 in, 3 out]
  n1139 = call "RSZVB Get IMOD Internal Combiner.vi"() -> ()  [unwired: 9 in, 3 out]
  n1140 = call "RSZVB Start IMOD Upper Tone Source Power Calibration.vi"() -> ()  [unwired: 10 in, 2 out]
  n1141 = call "RSZVB Get Noise Figure LO Oscillator.vi"() -> ()  [unwired: 9 in, 3 out]
  n1142 = call "RSZVB Get Virtual Transform Balanced Circuit Model.vi"() -> ()  [unwired: 9 in, 3 out]
  n1143 = call "RSZVB Get Virtual Transform Single Ended Port.vi"() -> ()  [unwired: 9 in, 3 out]
  n1144 = call "RSZVB Get Virtual Transform Ground Loop State.vi"() -> ()  [unwired: 9 in, 3 out]
  n1145 = call "RSZVB Set Virtual Transform Port Pair State.vi"() -> ()  [unwired: 10 in, 2 out]
  n1146 = call "RSZVB Load Port Pair Circuit Model Data.vi"() -> ()  [unwired: 10 in, 2 out]
  n1147 = call "RSZVB Set Sweep Time Auto.vi"() -> ()  [unwired: 10 in, 2 out]
  n1148 = call "RSZVB Get Noise Figure Calibration State.vi"() -> ()  [unwired: 9 in, 3 out]
  n1149 = call "RSZVB Get Sweep Count.vi"() -> ()  [unwired: 9 in, 3 out]
  n1150 = call "RSZVB Overwrite Noise Figure Channel Settings.vi"() -> ()  [unwired: 10 in, 2 out]
  n1151 = call "RSZVB Get Sweep Single - All Chans.vi"() -> ()  [unwired: 9 in, 3 out]
  n1152 = call "RSZVB Configure Trigger Settings.vi"() -> ()  [unwired: 10 in, 2 out]
  n1153 = call "RSZVB Set Trace Math Wave Quantity State.vi"() -> ()  [unwired: 10 in, 2 out]
  n1154 = call "RSZVB Get Common Mode Impedance.vi"() -> ()  [unwired: 9 in, 3 out]
  n1155 = call "RSZVB Get Port Groups Count.vi"() -> ()  [unwired: 9 in, 3 out]
  n1156 = call "RSZVB Get Calibration Kit User Connector Type With Label.vi"() -> ()  [unwired: 9 in, 3 out]
  n1157 = call "RSZVB Save Calibration Kit.vi"() -> ()  [unwired: 10 in, 2 out]
  n1158 = call "RSZVB Import Kit.vi"() -> ()  [unwired: 10 in, 2 out]
  n1159 = call "RSZVB Get Source Power Calibration Sensitivity Correction Range.vi"() -> ()  [unwired: 9 in, 3 out]
  n1160 = call "RSZVB Get Source Power Calibration Parameter Type.vi"() -> ()  [unwired: 9 in, 3 out]
  n1161 = call "RSZVB Get LN Preamplifier.vi"() -> ()  [unwired: 9 in, 3 out]
  n1162 = call "RSZVB Get External Signal Generator Output.vi"() -> ()  [unwired: 9 in, 3 out]
  n1163 = call "RSZVB Get IF Signal Port.vi"() -> ()  [unwired: 9 in, 3 out]
  n1164 = call "RSZVB Get External Signal Source.vi"() -> ()  [unwired: 9 in, 3 out]
  n1165 = call "RSZVB LO Source Calibration Stage 2.vi"() -> ()  [unwired: 10 in, 2 out]
  n1166 = call "RSZVB Get Simultaneous Measurement Minimum Frequency Offset Mode.vi"() -> ()  [unwired: 9 in, 3 out]
  n1167 = call "RSZVB Get Pulse Generator Single Period.vi"() -> ()  [unwired: 9 in, 3 out]
  n1168 = call "RSZVB Automatic Vector Mixer Calibration.vi"() -> ()  [unwired: 10 in, 2 out]
  n1169 = call "RSZVB Get Tolerance.vi"() -> ()  [unwired: 9 in, 3 out]
  n1170 = call "RSZVB Get Port Power Offset.vi"() -> ()  [unwired: 8 in, 4 out]
  n1171 = call "RSZVB Get Calibration Power Generator Offset.vi"() -> ()  [unwired: 9 in, 3 out]
  n1172 = call "RSZVB Get Power Calibration Method Source.vi"() -> ()  [unwired: 9 in, 3 out]
  n1173 = call "RSZVB Get Pulse Generator Master Channel.vi"() -> ()  [unwired: 9 in, 3 out]
  n1174 = call "RSZVB Get Pulse Train Segment Count.vi"() -> ()  [unwired: 9 in, 3 out]
  n1175 = call "RSZVB Set Chopped Pulse Profile Delay Increment.vi"() -> ()  [unwired: 10 in, 2 out]
  n1176 = call "RSZVB Get Advanced Power Transfer Model Frequency State.vi"() -> ()  [unwired: 9 in, 3 out]
  n1177 = call "RSZVB Get Converter Data Set Type.vi"() -> ()  [unwired: 9 in, 3 out]
  n1178 = call "RSZVB Get Port Transfer Model State.vi"() -> ()  [unwired: 9 in, 3 out]
  n1179 = call "RSZVB Set Port Waveguide Attenuator Offset.vi"() -> ()  [unwired: 10 in, 2 out]
  n1180 = call "RSZVB Set IMOD Receiver Port.vi"() -> ()  [unwired: 10 in, 2 out]
  n1181 = call "RSZVB Set IMOD Spectrum Measurement.vi"() -> ()  [unwired: 10 in, 2 out]
  n1182 = call "RSZVB Start IMOD Receive Port Source Power Calibration.vi"() -> ()  [unwired: 10 in, 2 out]
  n1183 = call "RSZVB Get Linearity Deviation Electrical Length.vi"() -> ()  [unwired: 9 in, 3 out]
  n1184 = call "RSZVB Get Fixed Frequency Signal.vi"() -> ()  [unwired: 9 in, 3 out]
  n1185 = call "RSZVB Get Fixed Frequency To Signal.vi"() -> ()  [unwired: 9 in, 3 out]
  n1186 = call "RSZVB Get Frequency High Accuracy.vi"() -> ()  [unwired: 9 in, 3 out]
  n1187 = call "RSZVB Get RF Image Frequency.vi"() -> ()  [unwired: 9 in, 3 out]
  n1188 = call "RSZVB Get Sweep Segments Count.vi"() -> ()  [unwired: 9 in, 3 out]
  n1189 = call "RSZVB Get Sweep Segment Stop Frequency.vi"() -> ()  [unwired: 9 in, 3 out]
  n1190 = call "RSZVB Get Sweep Segment Power.vi"() -> ()  [unwired: 9 in, 3 out]
  n1191 = call "RSZVB Get Sweep Segment Independent Bandwidth.vi"() -> ()  [unwired: 9 in, 3 out]
  n1192 = call "RSZVB Get Sweep Segment Selectivity.vi"() -> ()  [unwired: 9 in, 3 out]
  n1193 = call "RSZVB Get Sweep Segment Independent Time.vi"() -> ()  [unwired: 9 in, 3 out]
  n1194 = call "RSZVB Get Sweep Segment Triggering.vi"() -> ()  [unwired: 9 in, 3 out]
  n1195 = call "RSZVB Get Sweep Segment Bit Values.vi"() -> ()  [unwired: 6 in, 6 out]
  n1196 = call "RSZVB Query Sum Of Sweep Segments Time.vi"() -> ()  [unwired: 9 in, 3 out]
  n1197 = call "RSZVB Get Fixed Power.vi"() -> ()  [unwired: 9 in, 3 out]
  n1198 = call "RSZVB Get Signal Power Mode.vi"() -> ()  [unwired: 9 in, 3 out]
  n1199 = call "RSZVB Get Pulse Time Bandwidth.vi"() -> ()  [unwired: 9 in, 3 out]
  n1200 = call "RSZVB Get Pulse Evaluation Section Start.vi"() -> ()  [unwired: 9 in, 3 out]
  n1201 = call "RSZVB Get Pulse Shift Stimulus.vi"() -> ()  [unwired: 9 in, 3 out]
  n1202 = call "RSZVB Get Sweep Time Auto.vi"() -> ()  [unwired: 9 in, 3 out]
  n1203 = call "RSZVB Get Trace Math Wave Quantity State.vi"() -> ()  [unwired: 9 in, 3 out]
  n1204 = call "RSZVB Delete Group Of Measured Ports.vi"() -> ()  [unwired: 10 in, 2 out]
  n1205 = call "RSZVB Calibration Kit Catalog.vi"() -> ()  [unwired: 9 in, 3 out]
  n1206 = call "RSZVB Save Calibration Kit Ports.vi"() -> ()  [unwired: 10 in, 2 out]
  n1207 = call "RSZVB Additional Directory Calibration Kit.vi"() -> ()  [unwired: 10 in, 2 out]
  n1208 = call "RSZVB Get Source Power Calibration Paramater Attenuation.vi"() -> ()  [unwired: 9 in, 3 out]
  n1209 = call "RSZVB Set Pulse Modulator.vi"() -> ()  [unwired: 10 in, 2 out]
  n1210 = call "RSZVB Set Pulse Generator Train Period.vi"() -> ()  [unwired: 10 in, 2 out]
  n1211 = call "RSZVB Get Pulse Train Segments.vi"() -> ()  [unwired: 7 in, 5 out]
  n1212 = call "RSZVB Get Chopped Pulse Profile Delay Increment.vi"() -> ()  [unwired: 9 in, 3 out]
  n1213 = call "RSZVB Delete All Pulse Train Segments.vi"() -> ()  [unwired: 10 in, 2 out]
  n1214 = call "RSZVB Start IMOD Lower Upper Tone Ports Source Power Calibration.vi"() -> ()  [unwired: 10 in, 2 out]
  n1215 = call "RSZVB Set Frequency Conversion Mode.vi"() -> ()  [unwired: 10 in, 2 out]
  n1216 = call "RSZVB Set Frequency LO Conversion Factor.vi"() -> ()  [unwired: 10 in, 2 out]
  n1217 = call "RSZVB Get IMOD Receiver Port.vi"() -> ()  [unwired: 9 in, 3 out]
  n1218 = call "RSZVB Get IMOD Spectrum Measurement.vi"() -> ()  [unwired: 9 in, 3 out]
  n1219 = call "RSZVB Set Fixed Frequency Signal Stage 2.vi"() -> ()  [unwired: 10 in, 2 out]
  n1220 = call "RSZVB Get Source Power Calibration Paramater CW Power.vi"() -> ()  [unwired: 9 in, 3 out]
  n1221 = call "RSZVB Get Pulse Modulator.vi"() -> ()  [unwired: 9 in, 3 out]
  n1222 = call "RSZVB Application Example.vi"() -> ()  [unwired: 12 in, 4 out]
  n1223 = call "RSZVB Get Pulse Generator Train Period.vi"() -> ()  [unwired: 9 in, 3 out]
  n1224 = call "RSZVB Set Pulse Train Segment State.vi"() -> ()  [unwired: 10 in, 2 out]
  n1225 = call "RSZVB Save Pulse Train File.vi"() -> ()  [unwired: 10 in, 2 out]
  n1226 = call "RSZVB Get Fixed Frequency Signal Stage 2.vi"() -> ()  [unwired: 9 in, 3 out]
  n1227 = call "RSZVB Get Frequency LO Conversion Factor.vi"() -> ()  [unwired: 8 in, 4 out]
  n1228 = call "RSZVB Get Frequency Conversion Mode.vi"() -> ()  [unwired: 9 in, 3 out]
  n1229 = call "RSZVB Get Source Power Calibration Paramater CW Frequency.vi"() -> ()  [unwired: 9 in, 3 out]
  n1230 = call "RSZVB Get Source Power Calibration Paramater Timestamp.vi"() -> ()  [unwired: 9 in, 3 out]
  n1231 = call "RSZVB Revision Query.vi"() -> ()  [unwired: 8 in, 4 out]
  n1232 = call "RSZVB Error Query.vi"() -> ()  [unwired: 8 in, 4 out]
  n1233 = call "RSZVB Reset.vi"() -> ()  [unwired: 10 in, 2 out]
  n1234 = call "RSZVB State Checking.vi"() -> ()  [unwired: 10 in, 2 out]
  n1235 = call "RSZVB Write To Instrument.vi"() -> ()  [unwired: 10 in, 2 out]
  n1236 = call "RSZVB Close.vi"() -> ()  [unwired: 11 in, 1 out]
  n1237 = call "RSZVB Self-Test.vi"() -> ()  [unwired: 8 in, 4 out]
  n1238 = call "RSZVB Error Query (Multiple).vi"() -> ()  [unwired: 8 in, 4 out]
  n1239 = call "RSZVB Check Error.vi"() -> ()  [unwired: 10 in, 2 out]
  n1240 = call "RSZVB Option Checking.vi"() -> ()  [unwired: 10 in, 2 out]
  n1241 = call "RSZVB Read Instrument Data.vi"() -> ()  [unwired: 8 in, 4 out]
  n1242 = call "RSZVB Set Time Out.vi"() -> ()  [unwired: 10 in, 2 out]
  n1243 = call "RSZVB Get Time Out.vi"() -> ()  [unwired: 9 in, 3 out]
